vi "GDSLvIcon_DialogUpdateClass.vi"(1 "ClassPath(FilePath/ProjectTreePath/LvCLassRef)":variant, 2 "ClassName":string, 3 "Colors":T3={"Frame"=0, "Header Text Color"=0, "Header Background"=8453954, "BodyBackgroundPublic"=16121600, "BodyBackgroundProtected"=16777215, "BodyBackgroundPrivate"=16777215, "Body Text Color"=1, "Frame thickness"=1, "ProtectedPrivateSame"=TRUE, "Icon Header Size"=0, "Font Compression"=enum."Auto", "CapitalOnly"=TRUE}, 4 "AutoUpdate":bool, 5 "error in (no error)":errorcluster, 7 "HeaderToApply (take from VIRef or /use 2D-8bit header, Ignored if not wired)":variant, 9 "LibraryIcon":T1={"LibraryIcon"="Normal", "HeaderRows(1)"=0}) -> (15 "WholeIconOut":u8[][](array[numeric]) format="%x", 16 "Cancelled":bool, 17 "IconPictureOut":picture, 19 "error out":errorcluster)   [LabVIEW 2020]
uses:
  <resource>/Framework/Providers/Open_GDS/ClassProviders/Common/LvIcon_class/GDSLvIcon_ColorControl.ctl
  <resource>/Framework/Providers/Open_GDS/ClassProviders/Common/LvIcon_class/GDSLvIcon_ClassColorTypes.ctl
  <resource>/Framework/Providers/Open_GDS/ClassProviders/Common/LvIcon_class/GDSLvIcon_Type.ctl
  <resource>/Framework/Providers/Open_GDS/ClassProviders/Common/LvIcon_class/subvis/GDSLvIcon_TextDataType.ctl
  <resource>/Framework/Providers/Open_GDS/ClassProviders/Common/LvIcon_class/GDSLvIcon_WordCompressionType.ctl
  <resource>/Framework/Providers/Open_GDS/ClassProviders/Common/LvIcon_class/GDSLvIcon_TextAlignment.ctl
  <vilib>/event_ctls.llb/lveventtype.ctl
  <vilib>/picture/picture.llb/imagedata.ctl
  <resource>/Framework/Providers/Open_GDS/ClassProviders/Common/LvClass_class/GDSLvClass_IconSettingsType.ctl
panel:
  in  "NoSplitter":bool
  in  "_Back":bool
  in  "_OCR":bool
  in  "_MethodIconName":string caption="Body Text"
  in  "_DeleteIcon":bool
  in  "ClassIcon":u16(ring) items=["Normal", "Actor", "Message", "Interface", "Interface-I", "-", "Biosignal", "camera", "compression", "control dial", "database2", "GlobalVariable_48", "lc_testmode", "Lock-Lock-icon", "meter2", "motor_DC", "reset2", "signalProcessing", "SolidWorksModel", "sonar", "System", "Volts", "Warning2_32", "WarningOverlay", "-", "Add Icon..."]
  in  "_ClassIcon":string caption="Library icon"
  out "_Before":picture caption="Current"
  in  "_BodyColors":string caption="Body colors"
  in  "_Frame":string caption="Frame"
  in  "_Preview":string caption="Preview"
  in  "_RandomColorGeneration":string caption="Random color generation"
  in  "_Header":string caption="Header"
  in  "_Private":T2 caption="Private"
  in  "_Protected":T2 caption="Protected"
  in  "_Public":T2 caption="Public"
  in  "_Text":T2 caption="Text"
  in  "_ProtectedPrivateSame":bool=TRUE caption="Make Protected\nsame as Private"
  in  "_Dice":cluster{"Boolean 2":bool, "Dice 2":bool}
  out "_PrivateIcon":picture caption="Private icon"
  out "_ProtectedIcon":picture caption="Protected icon"
  out "_PublicIcon":picture caption="Public icon"
  out "_ClassIcon":picture caption="Library icon"
  out "_IconPreview":picture caption="Icon Preview"
  in  "_Frame":T2 caption="Frame"
  in  "_Thickness":u8=1 caption="Thickness (pixels)" min=1 max=3 step=1
  in  "_Rows":enum16{"1 Row", "2 Rows", "3 Rows"}(ring) caption="Rows"
  in  "_FontCompression":enum16{"Auto", "On", "Off"}(ring) caption="Font Compression"
  in  "_CapitalOnly":bool=TRUE caption="Force Capital Letters"
  in  "_Height":u8=9 caption="Height (pixels)" min=5 max=19
  in  "_Text":string="Endevo" caption="Text"
  in  "_HeaderBk":T2 caption="Background"
  in  "_HeaderText":T2 caption="Text"
  out "ClassName":string
  in  "_OK":bool
  out "Message":string
  in  "_Cancel":bool
  # "Backgrounds"
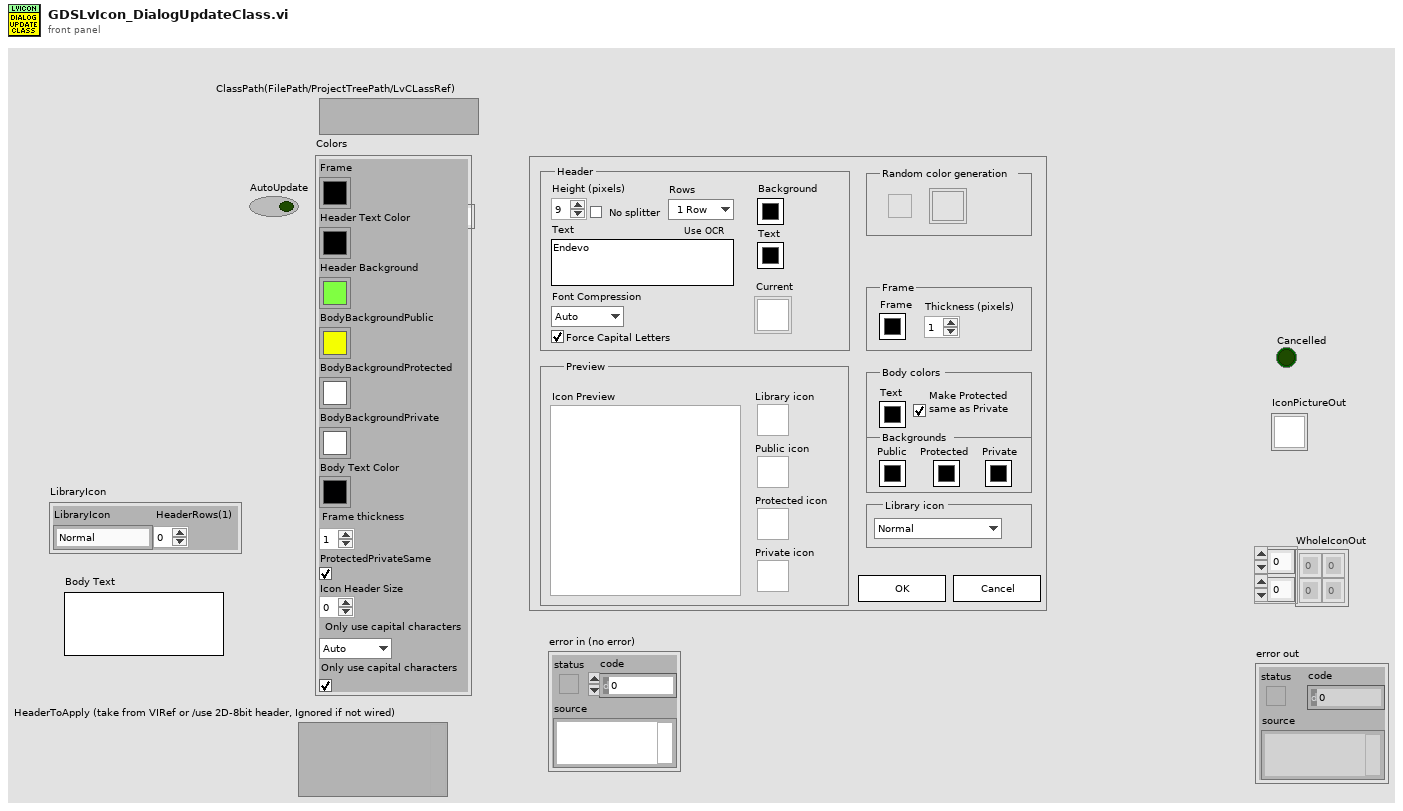
[diagram p1: front panel]
types:
  T1 = cluster{"LibraryIcon":string, "HeaderRows(1)":u8}
  T2 = typedef "GDSLvIcon_ColorControl.ctl" = cluster{"Decal":bool, "Color":u32}
  T3 = typedef "GDSLvIcon_ClassColorTypes.ctl" = cluster{"Frame":u32, "Header Text Color":u32, "Header Background":u32, "BodyBackgroundPublic":u32, "BodyBackgroundProtected":u32, "BodyBackgroundPrivate":u32, "Body Text Color":u32, "Frame thickness":u8, "ProtectedPrivateSame":bool, "Icon Header Size":u8, "Font Compression":enum16{"Auto", "On", "Off"}, "CapitalOnly":bool}
  T4 = typedef "GDSLvIcon_Type.ctl" = enum16{"LvClass", "Library", "X-Control", "LvInterface"}
  T5 = cluster{"Colors":T3, "LibraryIcon":cluster{"LibraryIcon":string, "HeaderRows(1)":u8}}
  T6 = cluster{"HText":string, "Library":refnum<vi>, "ClassItems":refnum<vi>[], "Header":u8[][], "ObjectBody":u8[][], "LvClassCreated":bool, "PreDefHeader":bool, "Type":T4, "DefaulIcons":i32, "AddIcon":i32, "NewIcon":string, "ClassBodyIcon":string, "ClassName":string, "FirstTime":bool, "_Back Colors":cluster{"_HeaderBK":u32, "_HeaderText":u32, "_Public":u32}, "IconIn":u8[][], "Cancelled":bool, "Splitter0px":bool}
  T7 = enum8{"Enabled", "Disabled", "Disabled and Grayed Out"}
  T8 = cluster{"Selection Start":u32, "Selection End":u32}
  T9 = typedef "GDSLvIcon_TextDataType.ctl" = cluster{"Text":string, "Allow Only Capital Chars":bool, "Compression":T10, "Alignment":T11}
  T10 = typedef "GDSLvIcon_WordCompressionType.ctl" = enum16{"Auto", "On", "Off"}
  T11 = typedef "GDSLvIcon_TextAlignment.ctl" = enum16{"Center", "Left", "Right"}
  T12 = typedef "lveventtype.ctl" = enum32{"Null", "Timeout", "Annotation Menu Selection", "Annotation Menu Selection?", "App Instance Close", "App Instance Close?", "Autoscale Range Change", "Bookmark Info Change", "Cell Edit", "Cell Edit?", "Cursor Grab", "Cursor Grab?", "Cursor Menu Selection", "Cursor Menu Selection?", "Cursor Move", "Cursor Release", "Data Change", "Direction Change", "Display State Change", "Drag Ended", "Drag Enter", "Drag Leave", "Drag Over", "Drag Source Update", "Drag Starting", "Drag Starting?", "Drop", "Exec State Change", "Key Down", "Key Down?", "Key Repeat", "Key Repeat?", "Key Up", "Listbox Double Click", "Menu Activation?", "Menu Selection (App)", "Menu Selection? (App)", "Menu Selection (User)", "Mouse Down", "Mouse Down?", "Mouse Enter", "Mouse Leave", "Mouse Move", "Mouse Up", "Mouse Wheel", "NI Security User Change (App)", "Pane Size", "Panel Close", "Panel Close?", "Panel Resize", "Plot Attribute Change", "Scale Range Change", "Shortcut Menu Activation?", "Shortcut Menu Selection (App)", "Shortcut Menu Selection? (App)", "Shortcut Menu Selection (User)", "Tree Double Click", "Tree Drag", "Tree Drag?", "Tree Drop", "Tree Drop?", "Tree Item Close", "Tree Item Close?", "Tree Item Open", "Tree Item Open?", "User Event", "Value Change"}
  T13 = typedef "GDSLvClass_IconSettingsType.ctl" = cluster{"Frame":u32, "Frame thickness":u8, "Header Background":u32, "Header Text":u32, "ColorPublic":u32, "ColorProtected":u32, "ColorPrivate":u32, "Body Text":u32, "ClassBodyIcon":string}
  T14 = typedef "imagedata.ctl" = cluster{"image type":i32, "image depth":i32, "image":u8[], "mask":u8[], "colors":u32[], "Rectangle":cluster{"left":i16, "top":i16, "right":i16, "bottom":i16}}
  T15 = enum32{"invalid lock state", "Not Locked", "Locked (No Password)", "Password-protected"}
  T16 = typedef "ColorControl.ctl" = cluster{"Decal":bool, "Color":u32}
  T17 = enum32{"invalid scope", "public", "private", "protected", "community"}
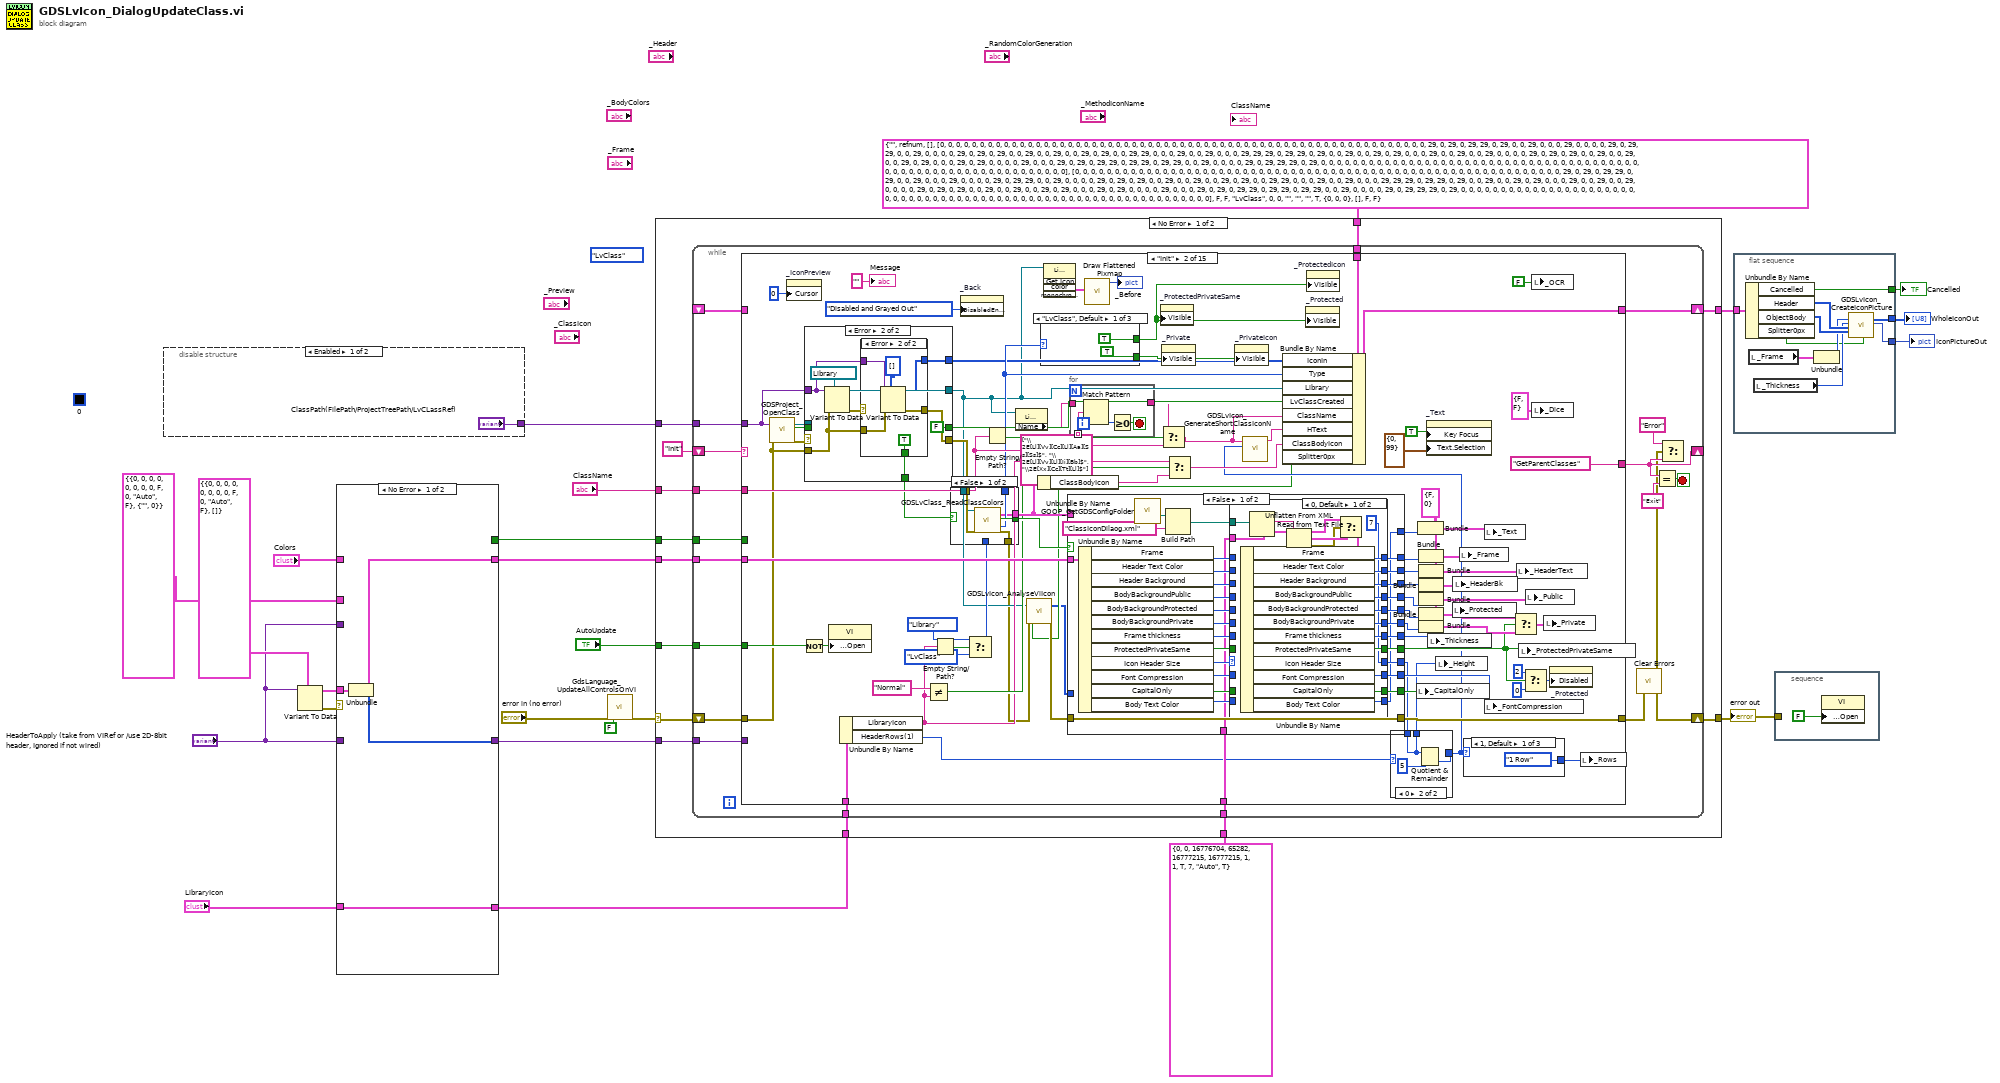
[diagram p0: block diagram]
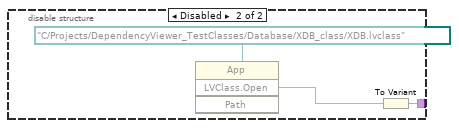
[diagram p2: hidden frame]
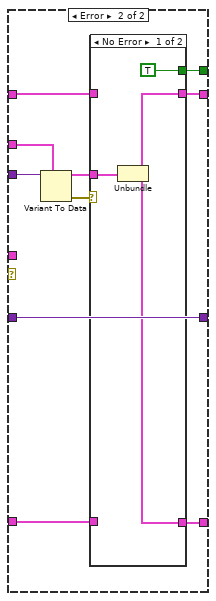
[diagram p3: hidden frame]
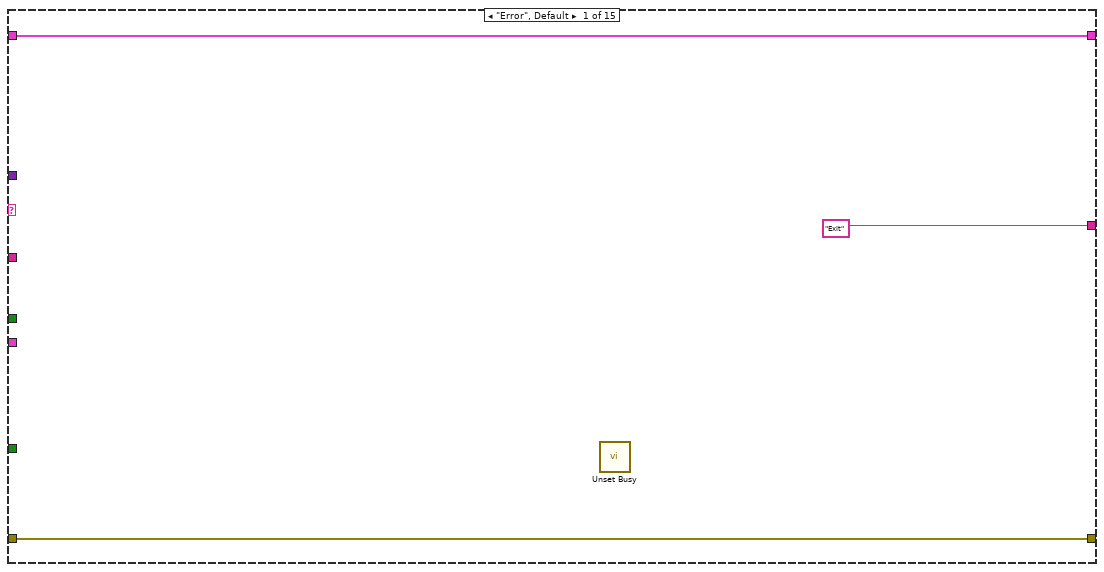
[diagram p5: hidden frame]
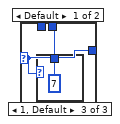
[diagram p7: hidden frame]
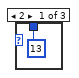
[diagram p8: hidden frame]
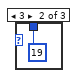
[diagram p9: hidden frame]
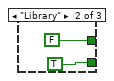
[diagram p10: hidden frame]
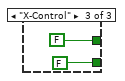
[diagram p11: hidden frame]
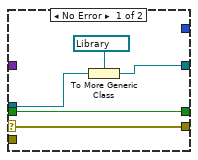
[diagram p12: hidden frame]
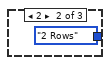
[diagram p14: hidden frame]
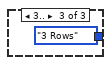
[diagram p15: hidden frame]
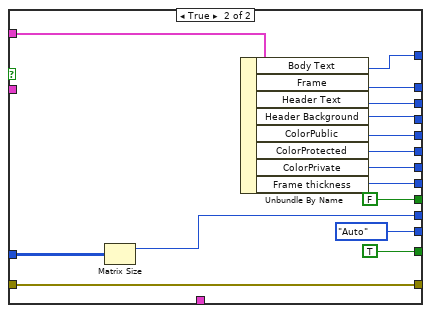
[diagram p17: hidden frame]
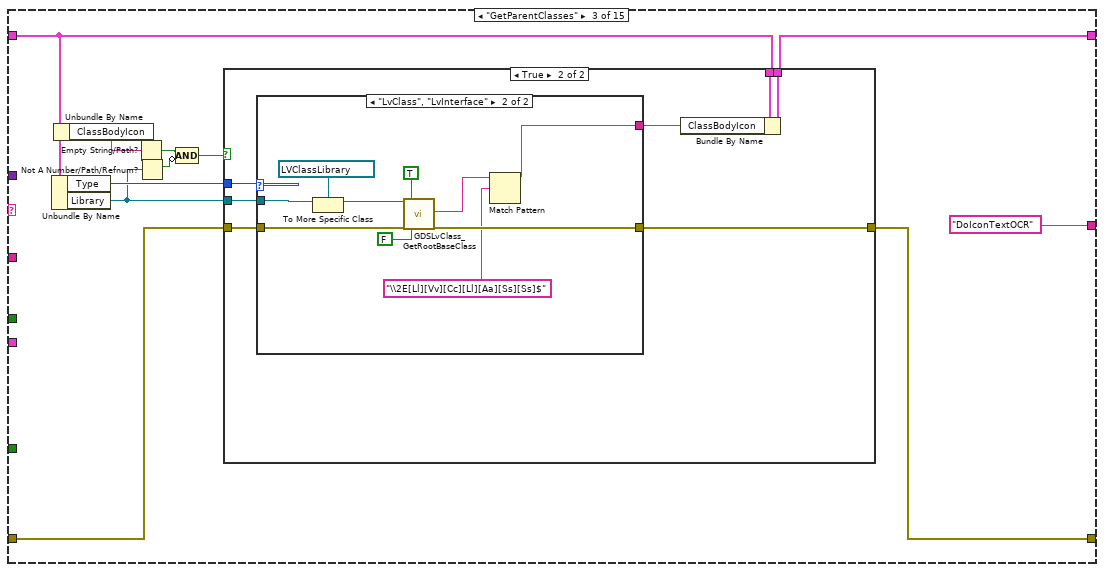
[diagram p18: hidden frame]
diagram:
  (unwired) GDSLvIcon_Type."LvClass" ("Type")
  (unwired) u32 0 ("Frame")
  n1 = disable-structure shown="Enabled" {
    disable-tunnel: ["ClassPath(FilePath/ProjectTreePath/LvCLassRef)" w28] -> w23
    frame Enabled {
    }
    frame Disabled {
      n2 = invoke class="App" method="LVClass.Open"("Path"=path "C:/Projects/DependencyViewer_TestClasses/Database/XDB_class/XDB.lvclass") -> ("LVClass.Open"=w26:refnum<vi>)  [unwired: 3 in, 3 out]
      n3 = To Variant(anything=w26) -> (Variant=w28:variant)
    }
  }
  n4 = Variant To Data(type=cluster{"Colors":T3, "TextOut":u8[][]} {"Colors"={"Frame"=0, "Header Text Color"=0, "Header Background"=0, "BodyBackgroundPublic"=0, "BodyBackgroundProtected"=0, "BodyBackgroundPrivate"=0, "Body Text Color"=0, "Frame thickness"=0, "ProtectedPrivateSame"=FALSE, "Icon Header Size"=0, "Font Compression"=enum."Auto", "CapitalOnly"=FALSE}, "TextOut"=[]} ("output cluster"), Variant="HeaderToApply (take from VIRef or /use 2D-8bit header, Ignored if not wired)") -> (data=w13:cluster{"Colors":T3, "TextOut":u8[][]}, error out=w14:errorcluster)  [unwired: 1 in]
  n5 = case shown="No Error" w14 {
    tunnel: w13 -> [w32 _]
    tunnel: [w31 w42] -> w12
    tunnel: "HeaderToApply (take from VIRef or /use 2D-8bit header, Ignored if not wired)" -> [_ w42]
    tunnel: "Colors" -> [_ w36]
    tunnel: [w30 w37] -> w10
    tunnel: "HeaderToApply (take from VIRef or /use 2D-8bit header, Ignored if not wired)" -> [_ w41]
    tunnel: T5 {"Colors"={"Frame"=0, "Header Text Color"=0, "Header Background"=0, "BodyBackgroundPublic"=0, "BodyBackgroundProtected"=0, "BodyBackgroundPrivate"=0, "Body Text Color"=0, "Frame thickness"=0, "ProtectedPrivateSame"=FALSE, "Icon Header Size"=0, "Font Compression"=enum."Auto", "CapitalOnly"=FALSE}, "LibraryIcon"={"LibraryIcon"="", "HeaderRows(1)"=0}} ("output cluster") -> [_ w40]
    tunnel: "LibraryIcon" -> [w29 w34]
    tunnel: [w29 w35] -> w6
    tunnel: [_ w33] -> w5
    frame No Error {
      n6 = Unbundle(w32) -> ("Colors"=w30:T3, "TextOut"=w31:u8[][])
    }
    frame Error {
      n7 = Variant To Data(type=w40, Variant=w41) -> (data=w38:T5, error out=w39:errorcluster)  [unwired: 1 in]
      n8 = case shown="No Error" w39 {
        tunnel: w38 -> [w46 _]
        tunnel: [w45 w48] -> w37
        tunnel: w36 -> [_ w48]
        tunnel: [w44 w47] -> w35
        tunnel: w34 -> [_ w47]
        tunnel: [TRUE _] -> w33
        frame No Error {
          n9 = Unbundle(w46) -> ("Colors"=w45:T3, "LibraryIcon"=w44:T1)
        }
        frame Error {
        }
      }
    }
  }
  n10 = call <resource>:"GdsLanguage_UpdateAllControlsOnVI.vi"("error in (no error)"="error in (no error)", "CreateLanguageFile(Use this to create a languageFile)"=FALSE) -> ("error out"=w16:errorcluster)  [unwired: 16 in, 1 out]
  n11 = case shown="No Error" w16 {
    selector: w16 -> [w60 w985]
    tunnel: [w59 w985] -> w19
    tunnel: w10 -> [w58 _]
    tunnel: "ClassName" -> [w57 _]
    tunnel: w23 -> [w56 _]
    tunnel: T6 {"HText"="", "Library"=refnum, "ClassItems"=[], "Header"=[[0, 0, 0, 0, 0, 0, 0, 0, 0, 0, 0, 0, 0, 0, 0, 0, 0, 0, 0, 0, 0, 0, 0, 0, 0, 0, 0, 0, 0, 0], [0, 0, 0, 0, 0, 0, 0, 0, 0, 0, 0, 0, 0, 0, 0, 0, 0, 0, 0, 0, 0, 0, 0, 0, 0, 0, 0, 0, 0, 0], [0, 29, 0, 29, 0, 29, 29, 0, 29, 0, 0, 29, 0, 0, 0, 29, 0, 0, 0, 0, 29, 0, 29, 29, 0, 0, 29, 0, 0, 0], [0, 29, 0, 29, 0, 29, 0, 0, 29, 0, 0, 29, 0, 0, 29, 0, 29, 0, 0, 29, 29, 0, 0, 0, 29, 0, 0, 29, 0, 0], [0, 29, 29, 29, 0, 29, 29, 0, 29, 0, 0, 29, 0, 0, 29, 0, 29, 0, 0, 0, 29, 0, 0, 29, 0, 0, 29, 0, 0, 0], [0, 29, 0, 29, 0, 29, 0, 0, 29, 0, 0, 29, 0, 0, 29, 0, 29, 0, 0, 0, 29, 0, 29, 0, 0, 0, 0, 29, 0, 0], [0, 29, 0, 29, 0, 29, 29, 0, 29, 29, 0, 29, 29, 0, 0, 29, 0, 0, 0, 0, 29, 0, 29, 29, 29, 0, 29, 0, 0, 0], [0, 0, 0, 0, 0, 0, 0, 0, 0, 0, 0, 0, 0, 0, 0, 0, 0, 0, 0, 0, 0, 0, 0, 0, 0, 0, 0, 0, 0, 0], [0, 0, 0, 0, 0, 0, 0, 0, 0, 0, 0, 0, 0, 0, 0, 0, 0, 0, 0, 0, 0, 0, 0, 0, 0, 0, 0, 0, 0, 0]], "ObjectBody"=[[0, 0, 0, 0, 0, 0, 0, 0, 0, 0, 0, 0, 0, 0, 0, 0, 0, 0, 0, 0, 0, 0, 0, 0, 0, 0, 0, 0, 0, 0], [0, 0, 0, 0, 0, 0, 0, 0, 0, 0, 0, 0, 0, 0, 0, 0, 0, 0, 0, 0, 0, 0, 0, 0, 0, 0, 0, 0, 0, 0], [0, 29, 0, 29, 0, 29, 29, 0, 29, 0, 0, 29, 0, 0, 0, 29, 0, 0, 0, 0, 29, 0, 29, 29, 0, 0, 29, 0, 0, 0], [0, 29, 0, 29, 0, 29, 0, 0, 29, 0, 0, 29, 0, 0, 29, 0, 29, 0, 0, 29, 29, 0, 0, 0, 29, 0, 0, 29, 0, 0], [0, 29, 29, 29, 0, 29, 29, 0, 29, 0, 0, 29, 0, 0, 29, 0, 29, 0, 0, 0, 29, 0, 0, 29, 0, 0, 29, 0, 0, 0], [0, 29, 0, 29, 0, 29, 0, 0, 29, 0, 0, 29, 0, 0, 29, 0, 29, 0, 0, 0, 29, 0, 29, 0, 0, 0, 0, 29, 0, 0], [0, 29, 0, 29, 0, 29, 29, 0, 29, 29, 0, 29, 29, 0, 0, 29, 0, 0, 0, 0, 29, 0, 29, 29, 29, 0, 29, 0, 0, 0], [0, 0, 0, 0, 0, 0, 0, 0, 0, 0, 0, 0, 0, 0, 0, 0, 0, 0, 0, 0, 0, 0, 0, 0, 0, 0, 0, 0, 0, 0], [0, 0, 0, 0, 0, 0, 0, 0, 0, 0, 0, 0, 0, 0, 0, 0, 0, 0, 0, 0, 0, 0, 0, 0, 0, 0, 0, 0, 0, 0]], "LvClassCreated"=FALSE, "PreDefHeader"=FALSE, "Type"=enum."LvClass", "DefaulIcons"=0, "AddIcon"=0, "NewIcon"="", "ClassBodyIcon"="", "ClassName"="", "FirstTime"=TRUE, "_Back Colors"={"_HeaderBK"=0, "_HeaderText"=0, "_Public"=0}, "IconIn"=[], "Cancelled"=FALSE, "Splitter0px"=FALSE} -> [w55 _]
    tunnel: T3 {"Frame"=0, "Header Text Color"=0, "Header Background"=16776704, "BodyBackgroundPublic"=65282, "BodyBackgroundProtected"=16777215, "BodyBackgroundPrivate"=16777215, "Body Text Color"=1, "Frame thickness"=1, "ProtectedPrivateSame"=TRUE, "Icon Header Size"=7, "Font Compression"=enum."Auto", "CapitalOnly"=TRUE} ("type") -> [w54 _]
    tunnel: "AutoUpdate" -> [w53 _]
    tunnel: w12 -> [w52 _]
    tunnel: w6 -> [w51 _]
    tunnel: w5 -> [w50 _]
    tunnel: [w49 _] -> w4
    frame No Error {
      n12 = while {
        shift-right: [w63] -> w59
        shift-left: w60 -> [w62]
        shift-right: [w64] -> _
        shift-left: "Init" -> [w67]
        shift-right: [w76] -> w49
        shift-left: _ -> [w75]
        tunnel: w58 -> [w74]
        tunnel: w57 -> [w73]
        tunnel: w56 -> [w72]
        tunnel: w55 -> [w71]
        tunnel: w54 -> [w70]
        tunnel: w53 -> [w69]
        tunnel: w52 -> [w68]
        tunnel: w51 -> [w66]
        tunnel: w50 -> [w65]
        stop <- w80 stop-if-true
        n13 = case shown="\"Init\"" w67 {
          selector: w67 -> [_ _ _ w327 w374 _ w480 _ _ w727 _ _ _ _ _]
          tunnel: w62 -> [w83 w118 w300 w333 w397 w431 w539 w556 w686 w733 w776 w784 w856 w896 w976]
          tunnel: [w83 w155 w299 w332 w397 w434 w526 w556 w686 w733 w775 w784 w846 w897 w970] -> w77
          tunnel: ["Exit" "GetParentClasses" "DoIconTextOCR" w336 "CheckPredefinedHeader" "UpdateIcons" w479 w557 w691 w726 w747 "UpdateClassDataIcon" "UpdateVIsIcons" "CloseRefs" "Exit"] -> w64
          tunnel: [w81 w156 w297 w328 w390 w433 w508 w554 w684 w723 w752 w787 w861 w899 w974] -> w76
          tunnel: w75 -> [w81 _ w298 w329 w372 w424 w487 w555 w685 w724 w752 w788 w860 w899 w974]
          tunnel: w74 -> [_ w162 _ _ _ _ _ w552 _ _ w773 _ _ _ _]
          tunnel: w73 -> [_ w153 _ _ _ _ _ _ _ _ _ _ _ _ _]
          tunnel: w72 -> [_ w121 _ _ _ _ _ _ _ _ _ _ _ _ _]
          tunnel: w71 -> [_ w157 _ _ _ _ _ _ _ _ _ _ _ _ _]
          tunnel: w70 -> [_ w149 _ _ _ _ _ _ _ _ _ _ _ _ _]
          tunnel: w69 -> [_ w148 _ _ _ _ _ w553 _ _ _ _ _ _ _]
          tunnel: w68 -> [_ _ _ _ _ w430 _ _ _ _ _ _ _ _ _]
          tunnel: w66 -> [_ w107 _ _ _ _ _ _ _ _ _ _ _ _ _]
          tunnel: w65 -> [_ _ _ _ _ _ _ w551 _ _ _ _ _ _ _]
          frame "Error", Default {
            n14 = call <vilib>:"Unset Busy.vi"() -> ()  [unwired: 11 in, 1 out]
          }
          frame "Init" {
            w134 = T2 {"Decal"=FALSE, "Color"=0} ("Frame")
            n15 = call <resource>:"GDSProject_OpenClass.vi"("ClassPath(FilePath/ProjectTreePath/LvCLassRef)"=w121, "error IO"=w118) -> ("LVClass.Open"=w117:refnum<vi>, "LvClassCreated"=w114:bool, "error out"=w120:errorcluster)  [unwired: 15 in]
            n16 = property on="_IconPreview" class="Pict"("Cursor"=0) -> ()  [unwired: 2 in, 2 out]
            n17 = Not(x=w148) -> (.not. x?=w147:bool)
            n18 = case shown="Error" w120 {
              selector: w120 -> [w196 _]
              tunnel: w121 -> [_ w199]
              tunnel: [w196 w201] -> w119
              tunnel: w118 -> [_ w200]
              tunnel: [w192 w204] -> w88
              tunnel: w117 -> [w193 _]
              tunnel: w114 -> [w195 _]
              tunnel: [w195 FALSE ("LvClassCreated")] -> w113
              tunnel: [_ w198] -> w95
              tunnel: [_ w197] -> w94
              frame No Error {
                n19 = To More Generic Class(target class=refnum<vi> refnum ("Library Refnum"), reference=w193) -> (generic class reference=w192:refnum<vi>)
              }
              frame Error {
                n20 = Variant To Data(error in=w200, type=refnum<vi> refnum ("Library Refnum"), Variant=w199) -> (data=w204:refnum<vi>, error out=w202:errorcluster)
                n21 = case shown="Error" w202 {
                  selector: w202 -> [w206 _]
                  tunnel: [w206 w209] -> w201
                  tunnel: w200 -> [_ w212]
                  tunnel: w199 -> [_ w210]
                  tunnel: [_ w208] -> w198
                  tunnel: [_ TRUE ("LvClassCreated")] -> w197
                  frame No Error {
                  }
                  frame Error {
                    n22 = Variant To Data(error in=w212, type=u8[][] [] ("TextOut"), Variant=w210) -> (data=w208:u8[][], error out=w209:errorcluster)
                  }
                }
              }
            }
            n23 = property class="VI"("Front Panel.Open"=w147) -> ()  [unwired: 2 in, 2 out]
            n24 = Unbundle By Name(w107) -> ("LibraryIcon"=w90:string, "HeaderRows(1)"=w102:u8)
            n25 = Not Equal?(x="Normal" ("LibraryIcon"), y=w90) -> (x != y?=w105:bool)
            n26 = Empty String/Path?(string/path=w90) -> (empty?=w91:bool)
            n27 = property on="_Back" class="Bool (strict)"("DisabledEnum"=T7."Disabled and Grayed Out" ("Disabled")) -> ()  [unwired: 2 in, 2 out]
            n28 = Select(t=GDSLvIcon_Type."Library" ("Type"), s=w91, f=GDSLvIcon_Type."LvClass" ("Type")) -> (s? t:f=w89:T4)
            n29 = case shown="False" w94 {
              tunnel: [w170 _] -> w150
              tunnel: w119 -> [w169 w172]
              tunnel: w88 -> [w168 _]
              tunnel: [w167 w171] -> w112
              tunnel: [w166 _] -> w108
              tunnel: [w165 w172] -> w87
              tunnel: w89 -> [_ w171]
              frame False {
                n30 = call <resource>:"GDSLvClass_ReadClassColors.vi"("Library Refnum"=w168, "error in (no error)"=w169) -> ("LvClassIconSettings"=w166:T13, "LvClassIconSettingsFound"=w170:bool, "Type"=w167:T4, "error out"=w165:errorcluster)  [unwired: 12 in, 2 out]
              }
              frame True {
              }
            }
            n31 = Empty String/Path?(string/path=w153) -> (empty?=w154:bool)
            n32 = property class="Library"(reference=w88) -> ("Name"=w110:string)  [unwired: 1 in, 2 out]
            n33 = call <resource>:"GDSLvIcon_AnalyseViIcon.vi"("ViRef/LvCLassRef/LvLibRef/ViPath/2D_Image"=w88, "error in (no error)"=w87) -> ("Splitter0px"=w85:bool, "HeaderIcon"=w84:u8[][], "error out"=w86:errorcluster)  [unwired: 4 in, 11 out]
            n34 = Unbundle By Name(w108) -> ("ClassBodyIcon"=w104:string)
            n35 = case shown="\"LvClass\", Default" w112 {
              tunnel: [TRUE FALSE FALSE] -> w115
              tunnel: [TRUE TRUE FALSE] -> w116
              frame "LvClass", Default {
              }
              frame "Library" {
              }
              frame "X-Control" {
              }
            }
            n36 = invoke class="Library" method="Get Icon"(reference=w88) -> ("color"=w122:T14)  [unwired: 4 in, 4 out]
            n37 = case shown="False" w150 {
              tunnel: [w244 w277] -> w124
              tunnel: w162 -> [w240 _]
              tunnel: [w239 w286] -> w146
              tunnel: [w238 w285] -> w138
              tunnel: [w237 w284] -> w137
              tunnel: [w236 w283] -> w136
              tunnel: [w235 w280] -> w161
              tunnel: [w234 enum16{"Auto", "On", "Off"}."Auto" ("Font Compression")] -> w160
              tunnel: [w233 TRUE ("CapitalOnly")] -> w159
              tunnel: [w222 FALSE ("ProtectedPrivateSame")] -> w128
              tunnel: [w221 w281] -> w133
              tunnel: [w220 w282] -> w135
              tunnel: w108 -> [_ w287]
              tunnel: w86 -> [w219 w276]
              tunnel: [w219 w276] -> w155
              tunnel: [w218 w279] -> w144
              tunnel: w149 -> [w216 _]
              tunnel: w84 -> [_ w278]
              frame False {
                n38 = Unbundle By Name(w240) -> ("Frame"=w232:u32, "Header Text Color"=w231:u32, "Header Background"=w230:u32, "BodyBackgroundPublic"=w229:u32, "BodyBackgroundProtected"=w228:u32, "BodyBackgroundPrivate"=w227:u32, "Frame thickness"=w226:u8, "ProtectedPrivateSame"=w225:bool, "Icon Header Size"=w245:u8, "Font Compression"=w224:enum16{"Auto", "On", "Off"}, "CapitalOnly"=w223:bool, "Body Text Color"=w217:u32)
                n39 = call <resource>:"GOOP_GetGDSConfigFolder.vi"() -> ("GDSFolderPath"=w243:path)
                n40 = Build Path(base path=w243, name or relative path="ClassIconDilaog.xml") -> (appended path=w241:path)
                n41 = case shown="0, Default" w245 {
                  selector: w245 -> [_ w275]
                  tunnel: [u8 7 ("Icon Header Size") w275] -> w244
                  tunnel: w241 -> [w263 _]
                  tunnel: [w261 w274] -> w239
                  tunnel: [w260 w273] -> w238
                  tunnel: [w259 w272] -> w237
                  tunnel: [w258 w271] -> w236
                  tunnel: [w257 w270] -> w220
                  tunnel: [w256 w269] -> w221
                  tunnel: [w255 w268] -> w235
                  tunnel: [w254 w267] -> w222
                  tunnel: [w253 w266] -> w234
                  tunnel: [w252 w265] -> w233
                  tunnel: w232 -> [_ w274]
                  tunnel: w231 -> [_ w273]
                  tunnel: w230 -> [_ w272]
                  tunnel: w229 -> [_ w271]
                  tunnel: w228 -> [_ w270]
                  tunnel: w227 -> [_ w269]
                  tunnel: w226 -> [_ w268]
                  tunnel: w225 -> [_ w267]
                  tunnel: w224 -> [_ w266]
                  tunnel: w223 -> [_ w265]
                  tunnel: w216 -> [w251 _]
                  tunnel: [w247 w264] -> w218
                  tunnel: w217 -> [_ w264]
                  frame 0, Default {
                    n42 = Read from Text File(file (use dialog)=w263) -> (text=w262:string)  [unwired: 3 in, 3 out]
                    n43 = Unflatten From XML(xml string=w262, type=w251) -> (value=w250:T3, error out=w249:errorcluster)  [unwired: 1 in]
                    n44 = Select(t=w251, s=w249, f=w250) -> (s? t:f=w248:T3)
                    n45 = Unbundle By Name(w248) -> ("Frame"=w261:u32, "Header Text Color"=w260:u32, "Header Background"=w259:u32, "BodyBackgroundPublic"=w258:u32, "BodyBackgroundProtected"=w257:u32, "BodyBackgroundPrivate"=w256:u32, "Frame thickness"=w255:u8, "ProtectedPrivateSame"=w254:bool, "Font Compression"=w253:enum16{"Auto", "On", "Off"}, "CapitalOnly"=w252:bool, "Body Text Color"=w247:u32)  [unwired: 1 out]
                  }
                  frame 1.. {
                  }
                }
              }
              frame True {
                n46 = Matrix Size(0:w278) -> (1:w277:i32)  [unwired: 1 out]
                n47 = Unbundle By Name(w287) -> ("Body Text"=w279:u32, "Frame"=w286:u32, "Header Text"=w285:u32, "Header Background"=w284:u32, "ColorPublic"=w283:u32, "ColorProtected"=w282:u32, "ColorPrivate"=w281:u32, "Frame thickness"=w280:u8)
              }
            }
            n48 = for {
              tunnel: string[] ["\\2E[Ll][Vv][Cc][Ll][Aa][Ss][Ss]$", "\\2E[Ll][Vv][Ll][Ii][Bb]$", "\\2E[Xx][Cc][Tt][Ll]$"] -> [w185] mode=indexing
              tunnel: [w182] -> w109
              tunnel: w110 -> [w181]
              stop <- w183 stop-if-true
              n49 = Match Pattern(string=w181, regular expression=w185) -> (before substring=w182:string, offset past match=w184:i32)  [unwired: 1 in, 2 out]
              n50 = Greater Or Equal To 0?(x=w184) -> (x >= 0?=w183:bool)
            }
            n51 = call <vilib>:"Draw Flattened Pixmap.vi"("image data"=w122) -> ("new picture"=→"_Before":picture)  [unwired: 8 in]
            n52 = property on="_ProtectedPrivateSame" class="Bool (strict)"("Visible"=w115) -> ()  [unwired: 2 in, 2 out]
            n53 = Select(t=w109, s=w154, f=w153) -> (s? t:f=w98:string)
            n54 = property on="_Private" class="Clust (strict)"("Visible"=w116) -> ()  [unwired: 2 in, 2 out]
            n55 = Select(t=w90, s=w105, f=w104) -> (s? t:f=w103:string)
            n56 = property on="_PrivateIcon" class="Pict"("Visible"=w116) -> ()  [unwired: 2 in, 2 out]
            n57 = property on="_Protected" class="Clust (strict)"("Visible"=w115) -> ()  [unwired: 2 in, 2 out]
            n58 = property on="_ProtectedIcon" class="Pict"("Visible"=w115) -> ()  [unwired: 2 in, 2 out]
            n59 = case shown="0" w102 {
              selector: w102 -> [w174 _]
              tunnel: [w174 w179] -> w101
              tunnel: w124 -> [_ w178]
              tunnel: [w173 w178] -> w99
              frame Default {
                n60 = case shown="1, Default" w174 {
                  tunnel: [u8 13 ("Icon Header Size") u8 19 ("Icon Header Size") u8 7 ("Icon Header Size")] -> w173
                  frame 2 {
                  }
                  frame 3 {
                  }
                  frame 1, Default {
                  }
                }
              }
              frame 0 {
                n61 = Quotient & Remainder(x=w178, y=u8 5) -> (floor(x/y)=w179:i32)  [unwired: 1 out]
              }
            }
            n62 = call <resource>:"GDSLvIcon_GenerateShortClassIconName.vi"("Rows(1)"=w101, "ClassName"=w98) -> ("ShortClassIconName"=w152:string)  [unwired: 9 in]
            n63 = Bundle By Name(cluster=w157, "IconIn"=w95, "Type"=w112, "Library"=w88, "LvClassCreated"=w113, "ClassName"=w98, "HText"=w152, "ClassBodyIcon"=w103, "Splitter0px"=w85) -> (w156:T6)
            n64 = local write "_CapitalOnly"(w159) -> ()
            n65 = Bundle(cluster=w134, "Color"=w144) -> (w143:T2)  [unwired: 1 in]
            n66 = Bundle(cluster=w134, "Color"=w146) -> (w145:T2)  [unwired: 1 in]
            n67 = Bundle(cluster=w134, "Color"=w138) -> (w142:T2)  [unwired: 1 in]
            n68 = Bundle(cluster=w134, "Color"=w137) -> (w141:T2)  [unwired: 1 in]
            n69 = Bundle(cluster=w134, "Color"=w136) -> (w140:T2)  [unwired: 1 in]
            n70 = Bundle(cluster=w134, "Color"=w135) -> (w139:T2)  [unwired: 1 in]
            n71 = Bundle(cluster=w134, "Color"=w133) -> (w132:T2)  [unwired: 1 in]
            n72 = property on="_Text" class="Str"("Key Focus"=TRUE, "Text.Selection"=T8 {"Selection Start"=0, "Selection End"=99}) -> ()  [unwired: 2 in, 2 out]
            n73 = local write "_Thickness"(w161) -> ()
            n74 = local write "_Height"(w99) -> ()
            n75 = local write "_Protected"(w139) -> ()
            n76 = local write "_HeaderBk"(w141) -> ()
            n77 = local write "_Frame"(w145) -> ()
            n78 = case shown="1, Default" w101 {
              tunnel: [enum16{"1 Row", "2 Rows", "3 Rows"}."1 Row" ("Rows") enum16{"1 Row", "2 Rows", "3 Rows"}."2 Rows" ("Rows") enum16{"1 Row", "2 Rows", "3 Rows"}."3 Rows" ("Rows")] -> w125
              frame 1, Default {
              }
              frame 2 {
              }
              frame 3.. {
              }
            }
            n79 = local write "_Text"(w143) -> ()
            n80 = local write "_FontCompression"(w160) -> ()
            n81 = Select(t=w139, s=w128, f=w132) -> (s? t:f=w158:T2)
            n82 = local write "_HeaderText"(w142) -> ()
            n83 = local write "_ProtectedPrivateSame"(w128) -> ()
            n84 = Select(t=u8 2 ("Disabled"), s=w128, f=u8 0 ("Disabled")) -> (s? t:f=w131:u8)
            n85 = local write "_Public"(w140) -> ()
            n86 = local write "_OCR"(FALSE ("_OCR")) -> ()
            n87 = local write "_Dice"(cluster{"Boolean 2":bool, "Dice":bool} {"Boolean 2"=FALSE, "Dice"=FALSE} ("Dice")) -> ()
            n88 = local write "_Private"(w158) -> ()
            n89 = property on="_Protected" class="Clust (strict)"("Disabled"=w131) -> ()  [unwired: 2 in, 2 out]
            n90 = local write "_Rows"(w125) -> ()
            "Message" <- "" ("Message")
          }
          frame "GetParentClasses" {
            n91 = Unbundle By Name(w298) -> ("Type"=w296:T4, "Library"=w292:refnum<vi>)
            n92 = Unbundle By Name(w298) -> ("ClassBodyIcon"=w295:string)
            n93 = Empty String/Path?(string/path=w295) -> (empty?=w294:bool)
            n94 = Not A Number/Path/Refnum?(number/path/refnum=w292) -> (NaN/Path/Refnum?=w293:bool)
            n95 = Compound Arithmetic op=AND(w294, invert w293) -> (w291:bool)
            n96 = case shown="True" w291 {
              tunnel: w292 -> [_ w305]
              tunnel: w300 -> [w302 w310]
              tunnel: [w302 w309] -> w299
              tunnel: w298 -> [w303 w308]
              tunnel: [w303 w307] -> w297
              tunnel: w296 -> [_ w304]
              frame False {
              }
              frame True {
                n97 = case shown="\"LvClass\", \"LvInterface\"" w304 {
                  tunnel: w305 -> [_ w314]
                  tunnel: w310 -> [w311 w321]
                  tunnel: [w311 w320] -> w309
                  tunnel: [_ w315] -> w306
                  frame Default {
                  }
                  frame "LvClass", "LvInterface" {
                    n98 = To More Specific Class(target class=refnum<vi> refnum ("LVClass.Open"), reference=w314) -> (specific class reference=w313:refnum<vi>)  [unwired: 1 in, 1 out]
                    n99 = call <resource>:"GDSLvClass_GetRootBaseClass.vi"("ViRef/Path,LvClassRef/Path"=w313, "error in (no error)"=w321, "Don'tOpenReference"=TRUE, "LimitToSpecificProviderTypeOfSameType(True)"=FALSE) -> ("ClassName"=w317:string, "error out"=w320:errorcluster)  [unwired: 9 in, 5 out]
                    n100 = Match Pattern(string=w317, regular expression="\\2E[Ll][Vv][Cc][Ll][Aa][Ss][Ss]$") -> (before substring=w315:string)  [unwired: 1 in, 3 out]
                  }
                }
                n101 = Bundle By Name(cluster=w308, "ClassBodyIcon"=w306) -> (w307:T6)
              }
            }
          }
          frame "DoIconTextOCR", "DoIconTextOCR:Idle" {
            n102 = Unbundle By Name(w329) -> ("FirstTime"=w326:bool, "ClassName"=w334:string, "HText"=w331:string, "IconIn"=w324:u8[][], "Library"=w323:refnum<vi>)  [unwired: 1 out]
            n103 = To Variant(anything=w324) -> (Variant=w322:variant)
            n104 = Not A Number/Path/Refnum?(number/path/refnum=w323) -> (NaN/Path/Refnum?=w325:bool)
            n105 = case shown="False" w325 {
              selector: w325 -> [w340 _]
              tunnel: [w347 w358] -> w335
              tunnel: w334 -> [w346 w358]
              tunnel: w333 -> [w345 w359]
              tunnel: [w344 w359] -> w332
              tunnel: w331 -> [w343 _]
              tunnel: w326 -> [w342 _]
              tunnel: w323 -> [w339 _]
              tunnel: w322 -> [w338 _]
              frame False {
                # "First Time and OCR Text Found"
                n106 = Select(t=w338, s=w340, f=w339) -> (s? t:f=w337:variant)
                n107 = call <resource>:"GDSLvIcon_AnalyseViIcon.vi"("ViRef/LvCLassRef/LvLibRef/ViPath/2D_Image"=w337, "DoATextOCR(False)"=TRUE, "error in (no error)"=w345) -> ("HeadText(OCR)"=w341:string, "error out"=w344:errorcluster)  [unwired: 3 in, 12 out]
                n108 = call <resource>:"GOOP_OCREvaluation.vi"("OcrText"=w341, "Viname"=w346) -> ("Match"=w349:bool)  [unwired: 9 in]
                n109 = Empty String/Path?(string/path=w341) -> (empty?=w352:bool)
                n110 = Compound Arithmetic op=AND(w342, invert w352) -> (w353:bool)
                n111 = local read "_OCR"() -> (w348:bool)
                n112 = And(x=w342, y=w349) -> (x .and. y?=w350:bool)
                n113 = Or(x=w350, y=w348) -> (x .or. y?=w351:bool)
                n114 = Select(t=w341, s=w351, f=w343) -> (s? t:f=w347:string)
                n115 = case shown="True" w353 {
                  tunnel: w349 -> [_ w355]
                  frame False {
                  }
                  frame True {
                    w356 = FALSE ("Boolean Text.Font:Bold")
                    n116 = property on="_OCR" class="Bool (strict)"("BoolText.FontBold"=w356, "BoolText.FontUnder"=w356, "Visible"=TRUE, "Value"=w355) -> ()  [unwired: 2 in, 2 out]
                  }
                }
              }
              frame True {
              }
            }
            n117 = local write "_Text"(w335) -> ()
            n118 = case shown="\"DoIconTextOCR:Idle\"" w327 {
              tunnel: ["UpdateIcons" "GetIcons"] -> w336
              frame "DoIconTextOCR:Idle" {
              }
              frame Default {
              }
            }
            n119 = Bundle By Name(cluster=w329, "FirstTime"=FALSE) -> (w328:T6)
          }
          frame "GetIcons", "GetIcons:AndSelect" {
            w383 = string[] ["Actor", "Message", "Interface", "Interface-I"] ("Strings []")
            n120 = call <resource>:"GOOP_GetProviderIniFilePath.vi"() -> ("ProviderMainFolder"=w387:path)  [unwired: 10 in, 1 out]
            n121 = Build Path(base path=w387, name or relative path="ClassBodyIcons") -> (appended path=w381:path)
            n122 = List Folder(path=w381) -> (filenames=w384:string[])  [unwired: 3 in, 3 out]
            n123 = for {
              shift-right: [w416] -> w382
              shift-left: w384 -> [w417]
              tunnel: w383 -> [w422] mode=indexing
              n124 = Concatenate Strings(w422, ".png" ("string")) -> (w420:string)
              n125 = To Lower Case(string=w420) -> (all lower case string=w418:string)
              n126 = To Lower Case(string=w417) -> (all lower case string=w419:string[])
              n127 = Search 1D Array(1D array=w419, element=w418) -> (index of element=w415:i32)  [unwired: 1 in]
              n128 = Delete From Array(array=w417, index=w415) -> (array with subset deleted=w416:string[])  [unwired: 1 in, 1 out]
            }
            n129 = Build Array (concatenate)("Normal", w383) -> (w385:string[])
            n130 = Equal?(x=w374, y="GetIcons:AndSelect") -> (x = y?=w370:bool)
            n131 = Unbundle By Name(w372) -> ("ClassBodyIcon"=w364:string, "NewIcon"=w371:string)
            n132 = for {
              tunnel: w382 -> [w410] mode=indexing
              tunnel: w381 -> [w409]
              shift-right: [w404] -> w378
              shift-left: string[] [] -> [w406]
              n133 = Build Path(base path=w409, name or relative path=w410) -> (appended path=w408:path)
              n134 = call <vilib>:"Get File Extension.vi"("file"=w408) -> ("filename without extension"=w405:string, "lowercase file extension"=w407:string)  [unwired: 6 in, 3 out]
              n135 = case shown="\"png\"" w407 {
                tunnel: w406 -> [w411 w414]
                tunnel: w405 -> [_ w413]
                tunnel: [w411 w412] -> w404
                frame Default {
                }
                frame "png" {
                  n136 = Build Array (concatenate)(w414, w413) -> (w412:string[])
                }
              }
            }
            n137 = To Lower Case(string=w364) -> (all lower case string=w362:string)
            n138 = Array Size(array=w378) -> (size(s)=w396:i32)
            n139 = Array Size(array=w385) -> (size(s)=w389:i32)
            n140 = Build Array (concatenate)("-", w378) -> (w393:string[])
            n141 = Greater Than 0?(x=w396) -> (x > 0?=w394:bool)
            n142 = Select(t=w393, s=w394, f=string[] []) -> (s? t:f=w380:string[])
            n143 = Build Array (concatenate)(w385, w380, string[] ["-", "Add Icon..."] ("f")) -> (w365:string[])
            n144 = Array Size(array=w365) -> (size(s)=w376:i32)
            n145 = case shown="Default" w362 {
              selector: w362 -> [_ w402]
              tunnel: w365 -> [_ w403]
              tunnel: [0 ("x") w401] -> w363
              frame "" {
              }
              frame Default {
                n146 = To Lower Case(string=w403) -> (all lower case string=w400:string[])
                n147 = Search 1D Array(1D array=w400, element=w402) -> (index of element=w401:i32)  [unwired: 1 in]
              }
            }
            n148 = Search 1D Array(1D array=w365, element=w371) -> (index of element=w369:i32)  [unwired: 1 in]
            n149 = Decrement(x=w376) -> (x-1=w375:i32)
            n150 = Select(t=w369, s=w370, f=w363) -> (s? t:f=w368:i32)
            n151 = Bundle By Name(cluster=w372, "AddIcon"=w375, "DefaulIcons"=w389) -> (w390:T6)
            n152 = Max & Min(x=0, y=w368) -> (max(x,y)=w366:i32)  [unwired: 1 out]
            n153 = Greater?(x=w366, y=w389) -> (0:w391:bool)
            n154 = property on="ClassIcon" class="Ring (strict)"("Strings []"=w365, "Value"=w366) -> ()  [unwired: 2 in, 2 out]
            n155 = property on="_DeleteIcon" class="Bool"("Visible"=w391) -> ()  [unwired: 2 in, 2 out]
          }
          frame "CheckPredefinedHeader" {
            n156 = Unbundle By Name(w424) -> ("Splitter0px"=w423:bool)
            n157 = Unbundle By Name(w424) -> ("IconIn"=w427:u8[][])
            n158 = Empty Array?(array=w427) -> (empty?=w428:bool)
            n159 = case shown="True" w428 {
              tunnel: [w438 w445] -> w436
              tunnel: [w439 w444] -> w435
              tunnel: w431 -> [w438 w443]
              tunnel: w430 -> [_ w442]
              tunnel: w427 -> [w440 _]
              tunnel: [_ TRUE ("PreDefHeader")] -> w426
              frame False {
                n160 = To Variant(anything=w440) -> (Variant=w439:variant)
              }
              frame True {
                n161 = Variant To Data(error in=w443, type=refnum<vi> refnum ("reference"), Variant=w442) -> (data=w444:refnum<vi>, error out=w445:errorcluster)
              }
            }
            n162 = case shown="No Error" w436 {
              selector: w436 -> [w466 _]
              tunnel: w435 -> [w464 _]
              tunnel: [w449 w470] -> w434
              tunnel: [w463 w473] -> w432
              tunnel: w431 -> [_ w469]
              tunnel: w430 -> [_ w472]
              tunnel: [w448 w468] -> w429
              tunnel: w426 -> [w448 _]
              tunnel: [w447 w467] -> w425
              tunnel: w423 -> [_ w467]
              frame No Error {
                w450 = T2 {"Decal"=FALSE, "Color"=0} ("Frame")
                n163 = call <resource>:"GDSLvIcon_AnalyseViIcon.vi"("ViRef/LvCLassRef/LvLibRef/ViPath/2D_Image"=w464, "error in (no error)"=w466) -> ("BodyTextColor"=w462:u32, "Splitter0px"=w447:bool, "HeaderTextColor"=w460:u32, "FrameColor"=w461:u32, "FrameThickness(1)"=w457:u32, "HeaderIcon"=w463:u8[][], "HeaderBkColor"=w459:u32, "BodyBkColor"=w458:u32, "error out"=w449:errorcluster)  [unwired: 4 in, 5 out]
                n164 = Array Size(array=w463) -> (size(s)=w465:i32[])
                n165 = Index Array(array=w465) -> (element=w456:i32)  [unwired: 1 in]
                n166 = Bundle(cluster=w450, "Color"=w462) -> (w454:T2)  [unwired: 1 in]
                n167 = Bundle(cluster=w450, "Color"=w461) -> (w455:T2)  [unwired: 1 in]
                n168 = Bundle(cluster=w450, "Color"=w460) -> (w453:T2)  [unwired: 1 in]
                n169 = Bundle(cluster=w450, "Color"=w459) -> (w452:T2)  [unwired: 1 in]
                n170 = Bundle(cluster=w450, "Color"=w458) -> (w451:T2)  [unwired: 1 in]
                n171 = local write "_Thickness"(w457) -> ()
                n172 = local write "_Height"(w456) -> ()
                n173 = local write "_HeaderBk"(w452) -> ()
                n174 = local write "_Frame"(w455) -> ()
                n175 = local write "_Text"(w454) -> ()
                n176 = local write "_HeaderText"(w453) -> ()
                n177 = local write "_Public"(w451) -> ()
              }
              frame Error {
                # "TBD"
                n178 = Variant To Data(error in=w469, type=u8[][] [] ("Header"), Variant=w472) -> (data=w473:u8[][], error out=w471:errorcluster)
                n179 = case shown="Error" w471 {
                  selector: w471 -> [w476 _]
                  tunnel: [w476 w477] -> w470
                  tunnel: w469 -> [_ w477]
                  tunnel: [TRUE ("PreDefHeader") _] -> w468
                  frame No Error {
                  }
                  frame Error {
                  }
                }
              }
            }
            n180 = Bundle By Name(cluster=w424, "Header"=w432, "PreDefHeader"=w429, "Splitter0px"=w425) -> (w433:T6)
          }
          frame "UpdateIcons", "UpdateIcons:GetClassChildren" {
            n181 = Unbundle By Name(w487) -> ("PreDefHeader"=w492:bool, "Header"=w491:u8[][], "Splitter0px"=w478:bool)  [unwired: 1 out]
            n182 = local read "_Text"() -> (w481:string)
            n183 = local read "_FontCompression"() -> (w537:enum16{"Auto", "On", "Off"})
            n184 = local read "_Frame"() -> (w505:T2)
            n185 = local read "_Thickness"() -> (w485:u8)
            n186 = local read "_CapitalOnly"() -> (w522:bool)
            n187 = local read "_Height"() -> (w529:u8)
            n188 = local read "_HeaderBk"() -> (w500:T2)
            n189 = Unbundle(w505) -> ("Color"=w506:u32)  [unwired: 1 out]
            n190 = local read "_HeaderText"() -> (w504:T2)
            n191 = local read "ClassIcon"() -> (w484:u16)
            n192 = local read "_Public"() -> (w502:T2)
            n193 = property on="ClassIcon" class="Ring (strict)"() -> ("Strings []"=w483:string[])  [unwired: 2 in, 2 out]
            n194 = case shown="\"Auto\", Default" w537 {
              tunnel: [enum16{"Auto", "On", "Off"}."Auto" ("Compression") enum16{"Auto", "On", "Off"}."Off" ("Compression") enum16{"Auto", "On", "Off"}."On" ("Compression")] -> w538
              frame "Auto", Default {
              }
              frame "Off" {
              }
              frame "On" {
              }
            }
            n195 = Bundle By Name(cluster=T9 {"Text"="", "Allow Only Capital Chars"=FALSE, "Compression"=enum."Auto", "Alignment"=enum."Center"} ("Text"), "Text"=w481, "Allow Only Capital Chars"=w522, "Compression"=w538) -> (w535:T9)
            n196 = Multiply(x=u8 2, y=w485) -> (x*y=w523:u8)
            n197 = Unbundle(w502) -> ("Color"=w501:u32)  [unwired: 1 out]
            n198 = Unbundle(w500) -> ("Color"=w499:u32)  [unwired: 1 out]
            n199 = Unbundle(w504) -> ("Color"=w503:u32)  [unwired: 1 out]
            n200 = case shown="Default" w484 {
              selector: w484 -> [_ w546]
              tunnel: w483 -> [_ w547]
              tunnel: [_ w545] -> w482
              frame 0 {
              }
              frame Default {
                n201 = Index Array(array=w547, index=w546) -> (element=w545:string)
              }
            }
            n202 = Subtract(x=32, y=w523) -> (x-y=w510:i32)
            n203 = call <resource>:"GDSLvIcon_GenerateIconText.vi"("Text"=w535, "TextPixelHeight(5-30)"=w529, "Foreground color"=w503, "Background color"=w499, "error in (no error)"=w539, "Text Pixel width(32-FrameThicknes*2))"=w510) -> ("TextOut"=w490:u8[][], "error out"=w534:errorcluster)  [unwired: 9 in, 3 out]
            n204 = local read "_Protected"() -> (w496:T2)
            n205 = local read "_Text"() -> (w498:T2)
            n206 = local read "_Private"() -> (w493:T2)
            n207 = Subtract(x=32, y=w529) -> (x-y=w533:i32)
            n208 = Select(t=w491, s=w492, f=w490) -> (s? t:f=w489:u8[][])
            n209 = Subtract(x=w533, y=w523) -> (x-y=w532:i32)
            n210 = Unbundle(w498) -> ("Color"=w497:u32)  [unwired: 1 out]
            n211 = case shown="True" w478 {
              tunnel: w532 -> [w541 w542]
              tunnel: [w540 w542] -> w509
              frame False {
                n212 = Decrement(x=w541) -> (x-1=w540:i32)
              }
              frame True {
              }
            }
            n213 = Unbundle(w496) -> ("Color"=w495:u32)  [unwired: 1 out]
            n214 = Unbundle(w493) -> ("Color"=w494:u32)  [unwired: 1 out]
            n215 = call <resource>:"GDSLvIcon_GenerateIconText.vi"("Text"=T9 {"Text"="PUBLIC", "Allow Only Capital Chars"=TRUE, "Compression"=enum."Auto", "Alignment"=enum."Center"}, "TextPixelHeight(5-30)"=w509, "Foreground color"=w497, "Background color"=w501, "Text Pixel width(32-FrameThicknes*2))"=w510) -> ("TextOut"=w520:u8[][], "error out"=w518:errorcluster)  [unwired: 10 in, 3 out]
            n216 = call <resource>:"GDSLvIcon_GenerateIconText.vi"("Text"=T9 {"Text"="PROTE-\nCTED", "Allow Only Capital Chars"=TRUE, "Compression"=enum."Auto", "Alignment"=enum."Center"}, "TextPixelHeight(5-30)"=w509, "Foreground color"=w497, "Background color"=w495, "Text Pixel width(32-FrameThicknes*2))"=w510) -> ("TextOut"=w515:u8[][], "error out"=w517:errorcluster)  [unwired: 10 in, 3 out]
            n217 = call <resource>:"GDSLvIcon_GenerateIconText.vi"("Text"=T9 {"Text"="PRIVATE", "Allow Only Capital Chars"=TRUE, "Compression"=enum."Auto", "Alignment"=enum."Center"}, "TextPixelHeight(5-30)"=w509, "Foreground color"=w497, "Background color"=w494, "Text Pixel width(32-FrameThicknes*2))"=w510) -> ("TextOut"=w488:u8[][], "error out"=w511:errorcluster)  [unwired: 10 in, 3 out]
            n218 = Unbundle By Name(w487) -> ("Type"=w486:T4)
            n219 = call <resource>:"GDSLvIcon_GenerateObjectIcon.vi"("HeaderColor"=w499, "BackgroundColor"=w501, "Height"=w509, "error in (no error)"=w534, "Type"=w486, "Width(30)"=w510, "ClassBodyIcon"=w482, "_Thickness"=w485) -> ("BodyIconOut"=w507:u8[][], "error out"=w527:errorcluster)  [unwired: 10 in]
            n220 = case shown="Default" w480 {
              tunnel: ["Idle" "GetClassChildren"] -> w479
              frame Default {
              }
              frame "UpdateIcons:GetClassChildren" {
              }
            }
            n221 = call <resource>:"GDSLvIcon_CreateIconPicture.vi"("FrameColor"=w506, "FrameThickness(1)"=w485, "HeaderIconIn"=w489, "BodyIconIn"=w507, "error in (no error)"=w527, "0px Splitter(False)"=w478) -> ("IconPictureOut"=→"_ClassIcon":picture, "LargeIconPictureOut(x6)"=→"_IconPreview":picture, "error out"=w526:errorcluster)  [unwired: 8 in, 3 out]
            n222 = call <resource>:"GDSLvIcon_CreateIconPicture.vi"("FrameColor"=w506, "FrameThickness(1)"=w485, "HeaderIconIn"=w489, "BodyIconIn"=w520, "error in (no error)"=w518, "0px Splitter(False)"=w478) -> ("IconPictureOut"=→"_PublicIcon":picture)  [unwired: 8 in, 5 out]
            n223 = call <resource>:"GDSLvIcon_CreateIconPicture.vi"("FrameColor"=w506, "FrameThickness(1)"=w485, "HeaderIconIn"=w489, "BodyIconIn"=w515, "error in (no error)"=w517, "0px Splitter(False)"=w478) -> ("IconPictureOut"=→"_ProtectedIcon":picture)  [unwired: 8 in, 5 out]
            n224 = call <resource>:"GDSLvIcon_CreateIconPicture.vi"("FrameColor"=w506, "FrameThickness(1)"=w485, "HeaderIconIn"=w489, "BodyIconIn"=w488, "error in (no error)"=w511, "0px Splitter(False)"=w478) -> ("IconPictureOut"=→"_PrivateIcon":picture)  [unwired: 8 in, 5 out]
            n225 = local write "NoSplitter"(w478) -> ()
            n226 = Bundle By Name(cluster=w487, "Header"=w489, "ObjectBody"=w507) -> (w508:T6)
          }
          frame "Idle" {
            (unwired) "Idle"
            n227 = case shown="False" w553 {
              tunnel: [w560 w681] -> w557
              tunnel: w555 -> [w559 w680]
              tunnel: [w558 w680] -> w554
              tunnel: w552 -> [_ w679]
              tunnel: w551 -> [_ w675]
              frame False {
                n228 = event shown="[16] \"_Thickness\", \"_Frame\": Value Change" {
                  selector: _ -> [_ _ _ _ _ _ _ _ _ _ _ _ _ _ _ _ _ _ _ _ _]
                  dyn-events: _ -> [_ _ _ _ _ _ _ _ _ _ _ _ _ _ _ _ _ _ _ _ _]
                  timeout: _ -> [_ _ _ _ _ _ _ _ _ _ _ _ _ _ _ _ _ _ _ _ _]
                  tunnel: ["Exit" "UpdateIcons" "DoIconTextOCR:Idle" "Idle" "Idle" "Idle" "Idle" "RandomColors" "UpdateIcons" w600 "GetIcons" "UpdateIcons" "Idle" "UpdateIcons" "UpdateIcons" "UpdateIcons" "UpdateIcons" "UpdateIcons" "UpdateIcons" "SaveSettings" "Exit"] -> w560
                  tunnel: w559 -> [w563 w567 w570 w574 w577 w580 w583 w585 w598 w605 w622 w623 w626 w634 w643 w646 w653 w655 w667 w668 w672]
                  tunnel: [w562 w566 w570 w574 w577 w580 w583 w585 w598 w605 w622 w623 w626 w634 w643 w646 w653 w655 w665 w668 w671] -> w558
                  event Panel Close? {
                    w561 = TRUE ("Discard?")
                    n229 = event-data() -> ()  [unwired: 1 in, 3 out]
                    n230 = Bundle By Name(cluster=w563, "Cancelled"=w561) -> (w562:T6)
                    n231 = event-data("Discard?"=w561) -> ()  [unwired: 1 in, 1 out]
                  }
                  event "_Text": Value Change; "_Text": Mouse Down {
                    n232 = event-data() -> ()  [unwired: 1 in, 1 out]
                    n233 = Bundle By Name(cluster=w567, "HText"="_Text") -> (w566:T6)
                  }
                  event "_OCR": Value Change {
                    w571 = FALSE ("Boolean Text.Font:Bold")
                    n234 = event-data() -> ()  [unwired: 1 in, 6 out]
                    n235 = property on="_OCR" class="Bool (strict)"("BoolText.FontBold"=w571, "BoolText.FontUnder"=w571) -> ()  [unwired: 2 in, 2 out]
                  }
                  event "_OCR": Mouse Enter {
                    w573 = TRUE ("Boolean Text.Font:Bold")
                    n236 = event-data() -> ()  [unwired: 1 in, 4 out]
                    n237 = property on="_OCR" class="Bool (strict)"("BoolText.FontBold"=w573, "BoolText.FontUnder"=w573) -> ()  [unwired: 2 in, 2 out]
                  }
                  event "_OCR": Mouse Leave {
                    w576 = FALSE ("Boolean Text.Font:Bold")
                    n238 = event-data() -> ()  [unwired: 1 in, 4 out]
                    n239 = property on="_OCR" class="Bool (strict)"("BoolText.FontBold"=w576, "BoolText.FontUnder"=w576) -> ()  [unwired: 2 in, 2 out]
                  }
                  event "_Dice": Mouse Enter {
                    n240 = event-data() -> ()  [unwired: 1 in, 1 out]
                    n241 = local write "_Dice"(cluster{"Boolean 2":bool, "Dice":bool} {"Boolean 2"=TRUE, "Dice"=FALSE} ("Dice")) -> ()
                  }
                  event "_Dice": Mouse Leave {
                    n242 = event-data() -> ()  [unwired: 1 in, 1 out]
                    n243 = local write "_Dice"(cluster{"Boolean 2":bool, "Dice":bool} {"Boolean 2"=FALSE, "Dice"=FALSE} ("Dice")) -> ()
                  }
                  event "_Dice": Value Change {
                    n244 = event-data() -> ()  [unwired: 1 in, 6 out]
                    n245 = local write "_Dice"(cluster{"Boolean 2":bool, "Dice":bool} {"Boolean 2"=TRUE, "Dice"=FALSE} ("Dice")) -> ()
                  }
                  event "_Back": Value Change {
                    w594 = T2 {"Decal"=FALSE, "Color"=0} ("Public")
                    n246 = event-data() -> ()  [unwired: 1 in, 6 out]
                    n247 = Unbundle By Name(w598) -> ("_Back Colors._HeaderBK"=w589:u32, "_Back Colors._HeaderText"=w587:u32, "_Back Colors._Public"=w588:u32)
                    n248 = Bundle By Name(cluster=w594, "Color"=u32 0) -> (w595:T2)
                    n249 = Bundle By Name(cluster=w594, "Color"=w589) -> (w593:T2)
                    n250 = Bundle By Name(cluster=w594, "Color"=w587) -> (w592:T2)
                    n251 = Bundle By Name(cluster=w594, "Color"=w588) -> (w591:T2)
                    n252 = property on="_Back" class="Bool (strict)"("DisabledEnum"=T7."Disabled and Grayed Out" ("Disabled")) -> ()  [unwired: 2 in, 2 out]
                    n253 = local write "_Text"(w595) -> ()
                    n254 = local write "_HeaderBk"(w593) -> ()
                    n255 = local write "_HeaderText"(w592) -> ()
                    n256 = local write "_Public"(w591) -> ()
                  }
                  event "ClassIcon": Value Change {
                    n257 = event-data() -> ("OldVal"=w599:u16)  [unwired: 1 in, 5 out]
                    n258 = Unbundle By Name(w605) -> ("DefaulIcons"=w604:i32, "AddIcon"=w603:i32)
                    n259 = Equal?(x="ClassIcon", y=w603) -> (x = y?=w601:bool)
                    n260 = case shown="False" w601 {
                      tunnel: w604 -> [w609 _]
                      tunnel: "ClassIcon" -> [w607 _]
                      tunnel: ["UpdateIcons" "AddIcon"] -> w600
                      tunnel: w599 -> [_ w610]
                      frame False {
                        n261 = Greater?(x=w607, y=w609) -> (0:w608:bool)
                        n262 = property on="_DeleteIcon" class="Bool"("Visible"=w608) -> ()  [unwired: 2 in, 2 out]
                      }
                      frame True {
                        n263 = property on="ClassIcon" class="Ring (strict)"("Value"=w610) -> ()  [unwired: 2 in, 2 out]
                      }
                    }
                  }
                  event "_DeleteIcon": Value Change {
                    n264 = event-data() -> ()  [unwired: 1 in, 1 out]
                    n265 = property on="ClassIcon" class="Ring (strict)"() -> ("Strings []"=w613:string[], "Value"=w614:u16)  [unwired: 2 in, 2 out]
                    n266 = call <resource>:"GOOP_GetProviderIniFilePath.vi"() -> ("ProviderMainFolder"=w615:path)  [unwired: 10 in, 1 out]
                    n267 = Index Array(array=w613, index=w614) -> (element=w618:string)
                    n268 = Build Path(base path=w615, name or relative path="ClassBodyIcons") -> (appended path=w620:path)
                    n269 = Concatenate Strings(w618, ".png" ("string")) -> (w619:string)
                    n270 = Build Path(base path=w620, name or relative path=w619) -> (appended path=w612:path)
                    n271 = Delete(path (use dialog)=w612) -> ()  [unwired: 4 in, 3 out]
                  }
                  event "_CapitalOnly", "_FontCompression": Value Change {
                    n272 = event-data() -> ()  [unwired: 1 in, 1 out]
                  }
                  event Mouse Enter; Mouse Leave {
                    n273 = event-data() -> ("Type"=w629:T12, "CtlRef"=w633:refnum<vi>)  [unwired: 1 in]
                    n274 = Equal?(x=w629, y=lveventtype."Mouse Enter") -> (x = y?=w627:bool)
                    n275 = property class="Clust (strict)"(reference=w633) -> (reference out=w632:refnum<vi>, "Value"=w631:T16)  [unwired: 1 in, 1 out]
                    n276 = Bundle By Name(cluster=w631, "Decal"=w627) -> (w630:T16)
                    n277 = property class="Clust (strict)"(reference=w632, "Value"=w630) -> ()  [unwired: 1 in, 2 out]
                  }
                  event Value Change {
                    n278 = event-data() -> ("NewVal"=w636:T2)  [unwired: 1 in]
                    n279 = local read "_ProtectedPrivateSame"() -> (w635:bool)
                    n280 = case shown="True" w635 {
                      tunnel: w636 -> [_ w638]
                      frame False {
                      }
                      frame True {
                        n281 = local write "_Private"(w638) -> ()
                        n282 = local write "_Protected"(w638) -> ()
                      }
                    }
                  }
                  event "_ProtectedPrivateSame": Value Change {
                    n283 = event-data() -> ()  [unwired: 1 in, 1 out]
                    n284 = local read "_Protected"() -> (w645:T2)
                    n285 = local write "_Private"(w645) -> ()
                    n286 = Select(t=u8 2 ("Disabled"), s="_ProtectedPrivateSame", f=u8 0 ("Disabled")) -> (s? t:f=w641:u8)
                    n287 = property on="_Protected" class="Clust (strict)"("Disabled"=w641) -> ()  [unwired: 2 in, 2 out]
                  }
                  event "_Rows": Value Change {
                    n288 = event-data() -> ()  [unwired: 1 in, 1 out]
                    n289 = case shown="\"1 Row\", Default" "_Rows" {
                      tunnel: [u8 7 ("Icon Header Size") u8 13 ("Icon Header Size") u8 19 ("Icon Header Size")] -> w648
                      frame "1 Row", Default {
                      }
                      frame "2 Rows" {
                      }
                      frame "3 Rows" {
                      }
                    }
                    n290 = local write "_Height"(w648) -> ()
                  }
                  event "_Thickness": Value Change {
                    n291 = event-data() -> ()  [unwired: 1 in, 1 out]
                  }
                  event "_Height": Value Change {
                    n292 = event-data() -> ()  [unwired: 1 in, 1 out]
                    n293 = Quotient & Remainder(x="_Height", y=u8 5) -> (floor(x/y)=w657:u8)  [unwired: 1 out]
                    n294 = case shown="1, Default" w657 {
                      tunnel: [enum16{"1 Row", "2 Rows", "3 Rows"}."1 Row" ("Rows") enum16{"1 Row", "2 Rows", "3 Rows"}."2 Rows" ("Rows") enum16{"1 Row", "2 Rows", "3 Rows"}."3 Rows" ("Rows")] -> w658
                      frame 1, Default {
                      }
                      frame 2 {
                      }
                      frame 3.. {
                      }
                    }
                    n295 = local write "_Rows"(w658) -> ()
                  }
                  event "NoSplitter": Value Change {
                    n296 = event-data() -> ()  [unwired: 1 in, 1 out]
                    n297 = Bundle By Name(cluster=w667, "Splitter0px"="NoSplitter") -> (w665:T6)
                  }
                  event "_OK": Value Change {
                    n298 = event-data() -> ()  [unwired: 1 in, 6 out]
                    n299 = call <vilib>:"Set Busy.vi"() -> ()  [unwired: 10 in, 2 out]
                  }
                  event "_Cancel": Value Change {
                    n300 = event-data() -> ()  [unwired: 1 in, 6 out]
                    n301 = Bundle By Name(cluster=w672, "Cancelled"="_Cancel") -> (w671:T6)
                  }
                }
              }
              frame True {
                n302 = Unbundle By Name(w679) -> ("Header Text Color"=w678:u32, "Header Background"=w677:u32)
                n303 = Equal?(x=w678, y=w677) -> (x = y?=w676:bool)
                n304 = And(x=w675, y=w676) -> (x .and. y?=w674:bool)
                n305 = case shown="False" w674 {
                  tunnel: ["RandomColors:UpdateIcons:GetClassChildren" "GetClassChildren"] -> w681
                  frame True {
                  }
                  frame False {
                  }
                }
              }
            }
          }
          frame "AddIcon" {
            n306 = call <resource>:"GOOP_GetProviderIniFilePath.vi"() -> ("ProviderMainFolder"=w688:path)  [unwired: 10 in, 1 out]
            n307 = Build Path(base path=w688, name or relative path="ClassBodyIcons") -> (appended path=w687:path)
            n308 = call "File Dialog"("prompt"="Select a PNG file to usa as a class icon.", "button label"="Add icon file", "pattern (all files)"="*.png") -> ("selected path"=w690:path, "cancelled"=w692:bool)  [unwired: 9 in, 2 out]
            n309 = case shown="False" w692 {
              tunnel: [w698 "Idle"] -> w691
              tunnel: w690 -> [w700 _]
              tunnel: w687 -> [w699 _]
              tunnel: w685 -> [w697 w714]
              tunnel: [w696 w714] -> w684
              frame False {
                n310 = Copy(10:w699, 11:w700) -> (0:w701:errorcluster)  [unwired: 3 in, 2 out]
                n311 = case shown="No Error" w701 {
                  tunnel: w700 -> [w705 w713]
                  tunnel: w699 -> [_ w710]
                  tunnel: ["GetIcons:AndSelect" "Idle"] -> w698
                  tunnel: w697 -> [w704 w707]
                  tunnel: [w703 w707] -> w696
                  frame No Error {
                    n312 = call <vilib>:"Get File Extension.vi"("file"=w705) -> ("filename without extension"=w702:string)  [unwired: 6 in, 4 out]
                    n313 = Bundle By Name(cluster=w704, "NewIcon"=w702) -> (w703:T6)
                  }
                  frame Error {
                    n314 = Strip Path(path=w713) -> (name=w712:string)  [unwired: 1 out]
                    n315 = Format Into String(format string="Error trying to copy the file: %s to this folder: %s" ("message"), w712, w710) -> (resulting string=w709:string)  [unwired: 2 in, 1 out]
                    n316 = One Button Dialog(message=w709) -> ()  [unwired: 1 in, 1 out]
                  }
                }
              }
              frame True {
              }
            }
          }
          frame "RandomColors", "RandomColors:UpdateIcons:GetClassChildren" {
            w731 = T2 {"Decal"=FALSE, "Color"=0} ("Public")
            w734 = u32[] [15007601, 14876576, 16751729, 15400704, 15507711, 16775072, 12713864, 12124142, 16776704, 16754080, 16752888, 16383904, 7667498, 16754986, 12112639, 3079936, 16776704, 16745561, 9341183, 16746660, 16773906, 2792191, 16762993, 5766954, 16318226, 15517125, 13290186, 10197915, 7442943, 11316396, 9743236, 16757617, 16767648, 6618880, 16711680, 16860, 16860, 16773906, 65421, 2789375, 13714175, 12827549, 10595204, 7641720, 6062466, 8025242, 11507131, 10386594, 786176, 8584960, 16318208, 16731648, 16755616, 16734715, 14399157, 16754801, 16714752, 10026888, 3524608]
            n317 = Random Number (0-1)() -> (number: 0 to 1=w742:dbl)
            n318 = Random Number (0-1)() -> (number: 0 to 1=w737:dbl)
            n319 = Array Size(array=w734) -> (size(s)=w736:i32)
            n320 = Build Array (concatenate)(w734, u32[] [10427904, 10442496, 10444544, 10452224, 10458112, 5927680, 3633920, 1351424, 35084, 40813, 16959, 19615, 1376393, 4194441, 10748084, 10420349, 7536704, 8978459, 5963776, 3882593, 4944486, 5204291, 7553536, 5263440, 4013373, 2763306, 6447714, 9540204, 6982244, 5470832, 6056066, 40848, 11010228]) -> (w740:u32[])
            n321 = Array Size(array=w740) -> (size(s)=w743:i32)
            n322 = property on="_Back" class="Bool (strict)"("DisabledEnum"=T7."Enabled" ("Disabled")) -> ()  [unwired: 2 in, 2 out]
            n323 = Multiply(x=w736, y=w737) -> (x*y=w738:dbl)
            n324 = Multiply(x=w743, y=w742) -> (x*y=w741:dbl)
            n325 = Round Toward -Infinity(1:w738) -> (0:w735:dbl)
            n326 = Round Toward -Infinity(1:w741) -> (0:w739:dbl)
            n327 = Index Array(array=w734, index=w735) -> (element=w719:u32)
            n328 = Index Array(array=w740, index=w739) -> (element=w718:u32)
            n329 = Greater?(x=w739, y=w736) -> ()  [unwired: 1 out]
            n330 = call <resource>:"GDSLvIcon_CalculateBrightness.vi"("RGB Color In"=w718) -> ("SuggestedTextColor"=w717:u32)  [unwired: 8 in, 2 out]
            n331 = feedback #1() -> (w722:u32)  [unwired: 1 in]
            n332 = feedback-in #1(w718) -> ()
            n333 = feedback #2() -> (w721:u32)  [unwired: 1 in]
            n334 = feedback-in #2(w717) -> ()
            n335 = feedback #3() -> (w720:u32)  [unwired: 1 in]
            n336 = feedback-in #3(w719) -> ()
            n337 = call <resource>:"GDSLvIcon_CalculateBrightness.vi"("RGB Color In"=w719) -> ("SuggestedTextColor"=w716:u32)  [unwired: 8 in, 2 out]
            n338 = Bundle By Name(cluster=w724, "_Back Colors._HeaderBK"=w722, "_Back Colors._HeaderText"=w721, "_Back Colors._Public"=w720) -> (w723:T6)
            n339 = case shown="Default" w727 {
              tunnel: ["UpdateIcons" "UpdateIcons:GetClassChildren"] -> w726
              frame Default {
              }
              frame "RandomColors:UpdateIcons:GetClassChildren" {
              }
            }
            n340 = Bundle By Name(cluster=w731, "Color"=w716) -> (w732:T2)
            n341 = Bundle By Name(cluster=w731, "Color"=w718) -> (w730:T2)
            n342 = Bundle By Name(cluster=w731, "Color"=w717) -> (w729:T2)
            n343 = Bundle By Name(cluster=w731, "Color"=w719) -> (w728:T2)
            n344 = local write "_HeaderBk"(w730) -> ()
            n345 = local write "_HeaderText"(w729) -> ()
            n346 = local write "_Text"(w732) -> ()
            n347 = local write "_Public"(w728) -> ()
          }
          frame "SaveSettings" {
            n348 = local read "_CapitalOnly"() -> (w768:bool)
            n349 = local read "_HeaderBk"() -> (w764:T2)
            n350 = local read "_Frame"() -> (w765:T2)
            n351 = local read "_Protected"() -> (w758:T2)
            n352 = local read "_Height"() -> (w770:u8)
            n353 = local read "_Thickness"() -> (w772:u8)
            n354 = Unbundle By Name(w764) -> ("Color"=w763:u32)
            n355 = Unbundle By Name(w758) -> ("Color"=w757:u32)
            n356 = Unbundle(w765) -> ("Color"=w766:u32)  [unwired: 1 out]
            n357 = local read "_Public"() -> (w760:T2)
            n358 = local read "_Private"() -> (w756:T2)
            n359 = local read "_FontCompression"() -> (w769:enum16{"Auto", "On", "Off"})
            n360 = local read "_HeaderText"() -> (w761:T2)
            n361 = local read "_ProtectedPrivateSame"() -> (w771:bool)
            n362 = local read "_Text"() -> (w754:T2)
            n363 = Unbundle By Name(w754) -> ("Color"=w753:u32)
            n364 = Unbundle By Name(w756) -> ("Color"=w755:u32)
            n365 = Unbundle By Name(w760) -> ("Color"=w759:u32)
            n366 = Unbundle By Name(w761) -> ("Color"=w762:u32)
            n367 = Unbundle By Name(w752) -> ("Library"=w751:refnum<vi>)
            n368 = Bundle By Name(cluster=w773, "Frame"=w766, "Header Text Color"=w762, "Header Background"=w763, "BodyBackgroundPublic"=w759, "BodyBackgroundProtected"=w757, "BodyBackgroundPrivate"=w755, "Frame thickness"=w772, "ProtectedPrivateSame"=w771, "Icon Header Size"=w770, "Font Compression"=w769, "CapitalOnly"=w768, "Body Text Color"=w753) -> (w767:T3)
            n369 = Not A Number/Path/Refnum?(number/path/refnum=w751) -> (NaN/Path/Refnum?=w750:bool)
            n370 = Flatten To XML(6:w767) -> (2:w777:string)
            n371 = call <resource>:"GOOP_GetGDSConfigFolder.vi"() -> ("GDSFolderPath"=w779:path)
            n372 = Build Path(base path=w779, name or relative path="ClassIconDilaog.xml") -> (appended path=w774:path)
            n373 = Select(t="Exit", s=w750, f="GetClassChildren") -> (s? t:f=w747:string)
            n374 = Write to Text File(file (use dialog)=w774, text=w777, error in=w776) -> (error out=w775:errorcluster)  [unwired: 1 in, 2 out]
          }
          frame "GetClassChildren" {
            n375 = Unbundle By Name(w788) -> ("Library"=w783:refnum<vi>)
            n376 = property class="Library"(reference=w783) -> ("Children[]"=w781:refnum<vi>[])  [unwired: 1 in, 2 out]
            n377 = Array Size(array=w781) -> (size(s)=w782:i32)
            n378 = Equal To 0?(x=w782) -> (x = 0?=w780:bool)
            n379 = case shown="False" w780 {
              tunnel: [w790 _] -> w786
              tunnel: w781 -> [w789 _]
              frame False {
                n380 = while {
                  shift-right: [w798] -> _
                  shift-left: w789 -> [w803]
                  shift-right: [w792] -> w790
                  shift-left: refnum<vi>[] [] -> [w793]
                  stop <- w799 stop-if-true
                  n381 = Delete From Array(array=w803, index=0) -> (deleted portion=w797:refnum<vi>, array with subset deleted=w801:refnum<vi>[])  [unwired: 1 in]
                  n382 = property class="ProjectItem"(reference=w797) -> (reference out=w795:refnum<vi>, "Type String"=w796:string)  [unwired: 1 in, 1 out]
                  n383 = case shown="\"Class Private Data\"" w796 {
                    tunnel: w795 -> [w804 w807 w812]
                    tunnel: [_ _ w814] -> w794
                    tunnel: w793 -> [w806 w809 w813]
                    tunnel: [w805 w808 w813] -> w792
                    frame Default {
                      n384 = Build Array (concatenate)(w806, w804) -> (w805:refnum<vi>[])
                    }
                    frame "Class Private Data" {
                      n385 = Build Array (concatenate)(w807, w809) -> (w808:refnum<vi>[])
                    }
                    frame "Folder" {
                      n386 = property class="ProjectItem"(reference=w812) -> (reference out=w810:refnum<vi>, error out=w811:errorcluster, "Children[]"=w814:refnum<vi>[])  [unwired: 1 in]
                      n387 = Close Reference(reference=w810, error in (no error)=w811) -> ()  [unwired: 1 out]
                    }
                  }
                  n388 = Build Array (concatenate)(w801, w794) -> (w798:refnum<vi>[])
                  n389 = Array Size(array=w798) -> (size(s)=w800:i32)
                  n390 = Equal To 0?(x=w800) -> (x = 0?=w799:bool)
                }
              }
              frame True {
              }
            }
            n391 = Bundle By Name(cluster=w788, "ClassItems"=w786) -> (w787:T6)
          }
          frame "UpdateClassDataIcon" {
            # "Updats the Icon layer info"
            n392 = Unbundle By Name(w860) -> ("Type"=w823:T4, "Library"=w821:refnum<vi>, "ClassItems"=w859:refnum<vi>[], "Header"=w817:u8[][], "ObjectBody"=w857:u8[][], "Splitter0px"=w815:bool)
            n393 = case shown="\"LvClass\"" w823 {
              tunnel: w859 -> [w864 w874]
              tunnel: [w864 w873] -> w858
              tunnel: w856 -> [w863 w872]
              tunnel: [_ w870] -> w849
              tunnel: [w863 w866] -> w829
              frame Default {
              }
              frame "LvClass" {
                n394 = Delete From Array(array=w874, index=0) -> (deleted portion=w871:refnum<vi>, array with subset deleted=w873:refnum<vi>[])  [unwired: 1 in]
                n395 = property class="ProjectItem"(reference=w871, error in=w872) -> (reference out=w869:refnum<vi>, error out=w867:errorcluster, "Reference"=w870:refnum<vi>)
                n396 = Close Reference(reference=w869, error in (no error)=w867) -> ()  [unwired: 1 out]
                n397 = call <resource>:"GDSError_ClearError.vi"("code"=1055, "error in (no error)"=w867) -> ("error out"=w866:errorcluster)  [unwired: 16 in, 1 out]
              }
            }
            n398 = case shown="\"LvClass\", Default" w823 {
              tunnel: [_ i32[] [5] ("codes")] -> w824
              tunnel: [w885 _] -> w822
              frame "LvClass", Default {
                n399 = local read "ClassIcon"() -> (w887:u16)
                n400 = property on="ClassIcon" class="Ring (strict)"() -> ("Strings []"=w886:string[])  [unwired: 2 in, 2 out]
                n401 = case shown="Default" w887 {
                  selector: w887 -> [_ w889]
                  tunnel: w886 -> [_ w890]
                  tunnel: [_ w888] -> w885
                  frame 0 {
                  }
                  frame Default {
                    n402 = Index Array(array=w890, index=w889) -> (element=w888:string)
                  }
                }
              }
              frame "X-Control" {
              }
            }
            n403 = local read "_HeaderText"() -> (w837:T2)
            n404 = local read "_Protected"() -> (w835:T2)
            n405 = local read "_Frame"() -> (w842:T2)
            n406 = local read "_Private"() -> (w838:T2)
            n407 = local read "_HeaderBk"() -> (w840:T2)
            n408 = local read "_Public"() -> (w833:T2)
            n409 = local read "_Thickness"() -> (w818:u8)
            n410 = local read "_Text"() -> (w832:T2)
            n411 = Unbundle(w842) -> ("Color"=w819:u32)  [unwired: 1 out]
            n412 = Unbundle By Name(w838) -> ("Color"=w836:u32)
            n413 = Unbundle By Name(w835) -> ("Color"=w834:u32)
            n414 = Unbundle By Name(w837) -> ("Color"=w839:u32)
            n415 = Unbundle By Name(w840) -> ("Color"=w841:u32)
            n416 = Unbundle By Name(w833) -> ("Color"=w831:u32)
            n417 = Unbundle By Name(w832) -> ("Color"=w830:u32)
            n418 = call <resource>:"GDSLvIcon_CreateIconPicture.vi"("FrameColor"=w819, "FrameThickness(1)"=w818, "HeaderIconIn"=w817, "BodyIconIn"=w857, "error in (no error)"=w829, "0px Splitter(False)"=w815) -> ("WholeIconOut"=w828:u8[][], "error out"=w820:errorcluster)  [unwired: 8 in, 4 out]
            n419 = Bundle By Name(cluster=T13 {"Frame"=0, "Frame thickness"=3, "Header Background"=8453954, "Header Text"=0, "ColorPublic"=16121600, "ColorProtected"=16777215, "ColorPrivate"=16777215, "Body Text"=0, "ClassBodyIcon"=""} ("LvClassIconSettings"), "ClassBodyIcon"=w822, "Body Text"=w830, "ColorPublic"=w831, "ColorProtected"=w834, "ColorPrivate"=w836, "Header Text"=w839, "Header Background"=w841, "Frame thickness"=w818, "Frame"=w819) -> (w843:T13)
            n420 = call <resource>:"GDSLvIcon_UpdateLibraryLayers.vi"("Library Refnum in"=w821, "FrameColor"=w819, "FrameThickness(1)"=w818, "HeaderIconIn"=w817, "error in (no error)"=w820, "0px Splitter(False)"=w815) -> ("error out"=w816:errorcluster)  [unwired: 12 in, 1 out]
            n421 = Reshape Array(w828, 1024 ("dimension size")) -> (w862:u8[])
            n422 = Bundle By Name(cluster=T14 {"image type"=0, "image depth"=8, "image"=[], "mask"=[], "colors"=[], "Rectangle"={"left"=0, "top"=0, "right"=32, "bottom"=32}} ("image data"), "image"=w862) -> (w825:T14)
            n423 = case shown="\"LvClass\"" w823 {
              tunnel: w820 -> [w875 w884]
              tunnel: [w875 w877] -> w850
              tunnel: w849 -> [_ w881]
              tunnel: w825 -> [_ w880]
              tunnel: w816 -> [_ _]
              frame Default {
              }
              frame "LvClass" {
                n424 = invoke class="VI" method="VI Icon.Set from Image Data"(reference=w881, error in=w884, "ImageData"=w880) -> (reference out=w883:refnum<vi>, error out=w882:errorcluster)  [unwired: 3 in, 4 out]
                n425 = invoke class="VI" method="Save.Instrument"(reference=w883, error in=w882) -> (reference out=w879:refnum<vi>, error out=w878:errorcluster)  [unwired: 4 in, 4 out]
                n426 = Close Reference(reference=w879) -> ()  [unwired: 1 in, 1 out]
                n427 = call <resource>:"GDSError_ClearError.vi"("code"=1055, "error in (no error)"=w878) -> ("error out"=w877:errorcluster)  [unwired: 16 in, 1 out]
              }
            }
            n428 = call <resource>:"GDSLvClass_StoreClassColors.vi"("Library Refnum"=w821, "LvClassIconSettings"=w843, "error in (no error)"=w850) -> ("Library Refnum"=w851:refnum<vi>, "error out"=w848:errorcluster)  [unwired: 15 in]
            n429 = Bundle By Name(cluster=w860, "ClassItems"=w858) -> (w861:T6)
            n430 = invoke class="Library" method="Set Icon"(reference=w851, error in=w848, "color"=w825) -> (reference out=w854:refnum<vi>, error out=w853:errorcluster)  [unwired: 2 in, 3 out]
            n431 = stacked-sequence {
              tunnel: w850 -> [_]
              frame #0 {
                n432 = local write "Message"("Updating Class template" ("Message")) -> ()
              }
            }
            n433 = invoke class="Library" method="Save"(reference=w854, error in=w853) -> (error out=w847:errorcluster)  [unwired: 2 in, 3 out]
            n434 = local write "Message"("Updating Object Icon" ("Message")) -> ()
            n435 = call <resource>:"GDSError_ClearError.vi"("code"=1055, "codes"=w824, "error in (no error)"=w847) -> ("error out"=w846:errorcluster)  [unwired: 15 in, 1 out]
          }
          frame "UpdateVIsIcons" {
            n436 = Unbundle By Name(w899) -> ("Library"=w900:refnum<vi>, "ClassItems"=w902:refnum<vi>[], "Splitter0px"=w893:bool)
            n437 = local read "_Text"() -> (w895:T2)
            n438 = Unbundle By Name(w895) -> ("Color"=w894:u32)
            n439 = Unbundle By Name(w899) -> ("Header"=w898:u8[][])
            n440 = for {
              N -> [w905]
              tunnel: w902 -> [w917] mode=indexing
              tunnel: w900 -> [w918]
              shift-right: [w911] -> w897
              shift-left: w896 -> [w912]
              tunnel: w898 -> [w910]
              tunnel: w894 -> [w904]
              tunnel: w893 -> [w903]
              i -> [w909]
              n441 = property class="ProjectItem"(reference=w917) -> ("Reference"=w915:refnum<vi>)  [unwired: 1 in, 2 out]
              n442 = invoke class="Library" method="Get Source Scope"(reference=w918, error in=w912, "SourceRef"=w917) -> (error out=w913:errorcluster, "GetSourceScope"=w914:T17)  [unwired: 2 in, 3 out]
              n443 = Not A Number/Path/Refnum?(number/path/refnum=w915) -> (NaN/Path/Refnum?=w916:bool)
              n444 = Increment(x=w909) -> (x+1=w908:i32)
              n445 = case shown="False" w916 {
                tunnel: w915 -> [w938 _]
                tunnel: w914 -> [w950 _]
                tunnel: w913 -> [w937 w969]
                tunnel: [w948 w969] -> w911
                tunnel: w910 -> [w947 _]
                tunnel: w904 -> [w921 _]
                tunnel: w903 -> [w919 _]
                frame False {
                  n446 = for {
                    tunnel: w938 -> [w963]
                    tunnel: string[] ["goop rules", "i love goteborg", "Endevo Knows Goop!"] -> [w962] mode=indexing
                    tunnel: w937 -> [w961]
                    tunnel: [w961] -> w936
                    w964 = FALSE ("Interactive")
                    n447 = invoke class="VI" method="Lock State.Set"(reference=w963, "lockState"=T15."Not Locked" ("Lock State"), "interactive"=w964, "password"=w962, "put in Cache"=w964) -> ()  [unwired: 2 in, 7 out]
                  }
                  n448 = case shown="\"public\", Default" w950 {
                    tunnel: [w966 w967 w968] -> w930
                    frame "public", Default {
                      n449 = local read "_Public"() -> (w966:T2)
                    }
                    frame "private" {
                      n450 = local read "_Private"() -> (w967:T2)
                    }
                    frame "protected" {
                      n451 = local read "_Protected"() -> (w968:T2)
                    }
                  }
                  n452 = call <resource>:"GDSLvIcon_AnalyseViIcon.vi"("ViRef/LvCLassRef/LvLibRef/ViPath/2D_Image"=w938, "error in (no error)"=w936) -> ("BodyTextColor"=w920:u32, "BodyIcon"=w952:u8[][], "BodyBkColor"=w951:u32, "error out"=w949:errorcluster)  [unwired: 4 in, 10 out]
                  n453 = Unbundle(w930) -> ("Color"=w927:u32)  [unwired: 1 out]
                  n454 = call <resource>:"GDSLvIcon_ReplaceIconColor.vi"("IconIn"=w952, "OldColor"=w951, "NewColor"=w927, "error in (no error)"=w949) -> ("IconOut"=w925:u8[][], "error out"=w923:errorcluster)  [unwired: 14 in]
                  n455 = Not Equal?(x=w920, y=w927) -> (x != y?=w926:bool)
                  n456 = case shown="True" w926 {
                    tunnel: w925 -> [w954 w960]
                    tunnel: [w954 w959] -> w924
                    tunnel: w923 -> [w953 w958]
                    tunnel: [w953 w957] -> w922
                    tunnel: w921 -> [_ w956]
                    tunnel: w920 -> [_ w955]
                    frame False {
                    }
                    frame True {
                      n457 = call <resource>:"GDSLvIcon_ReplaceIconColor.vi"("IconIn"=w960, "OldColor"=w955, "NewColor"=w956, "error in (no error)"=w958) -> ("IconOut"=w959:u8[][], "error out"=w957:errorcluster)  [unwired: 14 in]
                    }
                  }
                  n458 = local read "_Thickness"() -> (w940:u8)
                  n459 = local read "_Frame"() -> (w929:T2)
                  n460 = Unbundle(w929) -> ("Color"=w931:u32)  [unwired: 1 out]
                  n461 = call <resource>:"GDSLvIcon_CreateIconPicture.vi"("FrameColor"=w931, "FrameThickness(1)"=w940, "HeaderIconIn"=w947, "BodyIconIn"=w924, "error in (no error)"=w922, "0px Splitter(False)"=w919) -> ("WholeIconOut"=w944:u8[][], "error out"=w941:errorcluster)  [unwired: 8 in, 4 out]
                  n462 = Reshape Array(w944, 1024 ("dimension size")) -> (w942:u8[])
                  n463 = Bundle By Name(cluster=T14 {"image type"=0, "image depth"=8, "image"=[], "mask"=[], "colors"=[], "Rectangle"={"left"=0, "top"=0, "right"=32, "bottom"=32}} ("image data"), "image"=w942) -> (w945:T14)
                  n464 = invoke class="VI" method="VI Icon.Set from Image Data"(reference=w938, error in=w941, "ImageData"=w945) -> (reference out=w934:refnum<vi>, error out=w935:errorcluster)  [unwired: 3 in, 4 out]
                  n465 = call <resource>:"Scripting_SaveVi.vi"("ForceResaving(False)"=TRUE, "error in (no error)"=w935, "VIRefToSaveIn"=w934) -> ("error out"=w932:errorcluster, "VIRefToSaveOut"=w933:refnum<vi>)  [unwired: 7 in]
                  n466 = Close Reference(reference=w933, error in (no error)=w932) -> (error out=w948:errorcluster)
                }
                frame True {
                }
              }
              n467 = Format Into String(format string="Updating Icon %d of %d", w908, w905) -> (resulting string=w906:string)  [unwired: 2 in, 1 out]
              n468 = local write "Message"(w906) -> ()
            }
          }
          frame "CloseRefs" {
            n469 = Unbundle By Name(w974) -> ("LvClassCreated"=w972:bool, "Library"=w978:refnum<vi>, "ClassItems"=w977:refnum<vi>[])
            n470 = Close Reference(reference=w977, error in (no error)=w976) -> (error out=w975:errorcluster)
            n471 = case shown="True" w972 {
              tunnel: w978 -> [_ w984]
              tunnel: w975 -> [w981 w983]
              tunnel: [w981 w982] -> w971
              frame False {
              }
              frame True {
                n472 = Close Reference(reference=w984, error in (no error)=w983) -> (error out=w982:errorcluster)
              }
            }
            n473 = stacked-sequence {
              tunnel: w971 -> [w979]
              tunnel: [w980] -> _
              tunnel: [w979] -> w970
              frame #0 {
                n474 = call <vilib>:"Unset Busy.vi"("error in (no error)"=w979) -> ("error out"=w980:errorcluster)  [unwired: 10 in]
              }
            }
          }
        }
        n475 = call <vilib>:"Clear Errors.vi"("error in (no error)"=w77) -> ("error out"=w63:errorcluster)  [unwired: 5 in, 1 out]
        n476 = Equal?(x=w64, y="Exit") -> (x = y?=w80:bool)
        n477 = Select(t="Error", s=w63, f=w64) -> ()  [unwired: 1 out]
      }
    }
    frame Error {
    }
  }
  "error out" <- w19
  n478 = flat-sequence {
    tunnel: w4 -> [w995]
    tunnel: [w994] -> w3
    tunnel: [w988] -> w2
    tunnel: [w987] -> w1
    frame #0 {
      n479 = Unbundle By Name(w995) -> ("Cancelled"=w994:bool, "Header"=w993:u8[][], "ObjectBody"=w992:u8[][], "Splitter0px"=w986:bool)
      n480 = local read "_Frame"() -> (w991:T2)
      n481 = local read "_Thickness"() -> (w990:u8)
      n482 = Unbundle(w991) -> ("Color"=w989:u32)  [unwired: 1 out]
      n483 = call <resource>:"GDSLvIcon_CreateIconPicture.vi"("FrameColor"=w989, "FrameThickness(1)"=w990, "HeaderIconIn"=w993, "BodyIconIn"=w992, "0px Splitter(False)"=w986) -> ("WholeIconOut"=w988:u8[][], "IconPictureOut"=w987:picture)  [unwired: 9 in, 4 out]
    }
  }
  n484 = stacked-sequence {
    tunnel: w19 -> [_]
    frame #0 {
      n485 = property class="VI"("Front Panel.Open"=FALSE ("Front Panel Window:Open")) -> ()  [unwired: 2 in, 2 out]
    }
  }
  "Cancelled" <- w3
  "WholeIconOut" <- w2
  "IconPictureOut" <- w1
